vi "XLIN1.7-2048SQ TE0_Target.vi"() -> ()   [LabVIEW 2018]
uses:
  <vilib>/Platform/TimedLoop/XDataNode/timing_clust.ctl
  <vilib>/Platform/TimedLoop/XDataNode/nitl_modes.ctl
  <vilib>/Platform/TimedLoop/XDataNode/wakeup.ctl
  <vilib>/rvi/eio/common/nirviEmuTemplateMethod_errors.vi
  <vilib>/rvi/Emulation/niFpgaGetClockAttributes.vi
  <vilib>/rvi/Emulation/niFpgaSctlEmulationGetInTimedLoop.vi
  <vilib>/rvi/Emulation/niFpgaEmulationReportErrorSimple.vi
  <vilib>/rvi/Emulation/niFpgaProcessEmulError.vi
  <vilib>/rvi/Emulation/niFpgaCriticalErrorInLSC.vi
  <vilib>/rvi/interface/RandomDataEmulation/niFpgaRandomDataHandleErrors.vi
  <vilib>/eio/EIONode/EIONode.xnode
  <vilib>/Platform/TimedLoop/XDataNode/XDataNode.xnode
  <vilib>/rvi/DataTransferAndStorage/Container/XNode/niFpgaContainer.xnode
  <vilib>/rvi/interface/RandomDataEmulation/nirviRandomDataFpgaReadWriteTemplate.vi
  <vilib>/Platform/TimedLoop/XDataNode/XDNodeRunTimeDep.lvlib
panel:
  in  "SetFull":bool
  in  "GetCapture":bool
  in  "FIFO Enable = 0":u8
  in  "Ticks Reset = 7":u8=7
  in  "Tick Before Low CS":u64=1
  in  "Ticks After End Readout >0":u64=1
  in  "Ticks After ADC":u64
  in  "Stop FIFO Frame":u8=7
  in  "Output Data _ADCCLK(F) = 7":u8=7
  in  "True CDSCLK2 Stop = 5":u8=1
  in  "True CDSCLK2 Start = 4":u8
  in  "Ticks After Start Readout":u64=4
  in  "Ticks After Start Integration":u64
  in  "Ticks After Reset":u64
  in  "Ticks After Bot >0":u64=64
  in  "Ticks After Top >0":u64=64
  in  "Supply Select":u8(ring) items=["Local", "External"]
  in  "Counter R&F CLK_2 = 4":u8=4
  in  "F(F)/R(T)_CmAD":bool
  in  "Output Data _ADCCLK(T) = 3":u8=3
  in  "True ADCCLK Stop = 4":u8=4
  in  "True ADCCLK Start = 1":u8=1
  in  "Counter R&F CLK_1 = 7":u8=7
  in  "Falling CLK_2 = 2":u8=2
  in  "Rising CLK_2 = 1":u8=1
  in  "Falling CLK_1 = 1":u8=1
  in  "Rising CLK_1 = 0":u8
  in  "Counter R CLK = 2":u8=2
  in  "ResetFrame":bool
  in  "Data End Readout":u8[](array[numeric])=[0, 5, 1, 0, 0]
  in  "Command End Readout":u8[](array[numeric])=[8, 4, 2, 0, 0]
  in  "Data Start Readout":u8[](array[numeric])=[0, 0, 1, 11, 1, 0, 0, 0, 0, 6, 0, 0, 15, 0, 1, 3, 5, 13, 13, 0]
  in  "Command Start Readout":u8[](array[numeric])=[8, 4, 2, 2, 2, 2, 9, 2, 2, 2, 2, 2, 2, 1, 1, 1, 1, 1, 1, 0]
  in  "Data Start Integration":u8[](array[numeric])=[0, 0, 0, 1, 1, 0, 0, 0, 5, 1, 0, 0, 0, 0, 0, 0, 0, 0, 0, 0, 3, 1, 0, 0, 1, 5, 1, 0, 0, 1, 3, 1, 0, 0, 1, 3, 1, 0, 0, 1, 11, 1, 11, 0, 1, 11, 1, 3, 0, 0, 0]
  in  "Command Start Integration":u8[](array[numeric])=[8, 4, 2, 2, 2, 2, 9, 2, 2, 2, 2, 2, 0, 0, 0, 0, 0, 8, 4, 2, 2, 2, 2, 9, 2, 2, 2, 2, 9, 2, 2, 2, 2, 9, 2, 2, 2, 2, 9, 2, 2, 2, 2, 9, 2, 2, 2, 2, 9, 0, 0]
  in  "Data Reset":u8[](array[numeric])=[0, 0, 0, 5, 0, 0, 0, 0]
  in  "Command Reset":u8[](array[numeric])=[8, 4, 2, 2, 2, 2, 9, 0]
  in  "IN1":bool
  in  "IN2":bool
  in  "RS":bool
  in  "1032 pixels":u16=1032
  in  "Pixel (n-3) = 3":u16=3
  in  "R MCLK = 2":u16=2
  in  "Command array":bool[](array[boolean])=[FALSE, FALSE, FALSE, FALSE, FALSE, FALSE, FALSE, FALSE, FALSE, FALSE, FALSE, FALSE, FALSE, FALSE, FALSE, FALSE, FALSE]
  in  "Read(T)/Write(F)":bool
  in  "Enum":T1(ring)=enum."GREEN PGA"
  in  "Write Data":bool[](array[boolean])=[FALSE, FALSE, FALSE, FALSE, FALSE, FALSE, FALSE, FALSE, FALSE]
  out "READ":bool[](array[boolean])
  in  "Конфигурация":bool
  out "FrameIsDone":bool
  in  "NumberOfAddFIFO":u16=2064
  in  "7..0(F)/0..7(T)":bool
  out "FIFOCounter":u16
  in  "Data CSBot":u8[](array[numeric])=[0, 9, 8, 11, 0, 6, 0, 2, 11, 0, 8, 0, 0, 0, 0, 9, 1, 3, 11, 7, 15, 15, 5, 15, 0, 1, 15, 15, 5, 8, 5, 2, 3, 0, 8, 2, 3, 3, 3, 3, 3, 3, 3, 2, 0]
  in  "Автомат":bool
  in  "Data CSTop":u8[](array[numeric])=[0, 9, 12, 11, 0, 6, 0, 2, 11, 0, 8, 0, 0, 0, 0, 9, 1, 3, 3, 7, 15, 15, 5, 15, 0, 1, 15, 15, 5, 8, 5, 2, 3, 0, 8, 2, 3, 3, 3, 3, 3, 3, 3, 2, 0]
  in  "Command CS":u8[](array[numeric])=[8, 4, 2, 2, 2, 2, 2, 2, 2, 2, 2, 2, 2, 2, 2, 2, 2, 2, 2, 2, 2, 2, 2, 2, 2, 2, 2, 2, 2, 2, 2, 2, 2, 8, 4, 1, 1, 1, 1, 1, 1, 1, 1, 1, 0]
  in  "Stop_FPGA":bool
  in  "SetPreCapture":bool
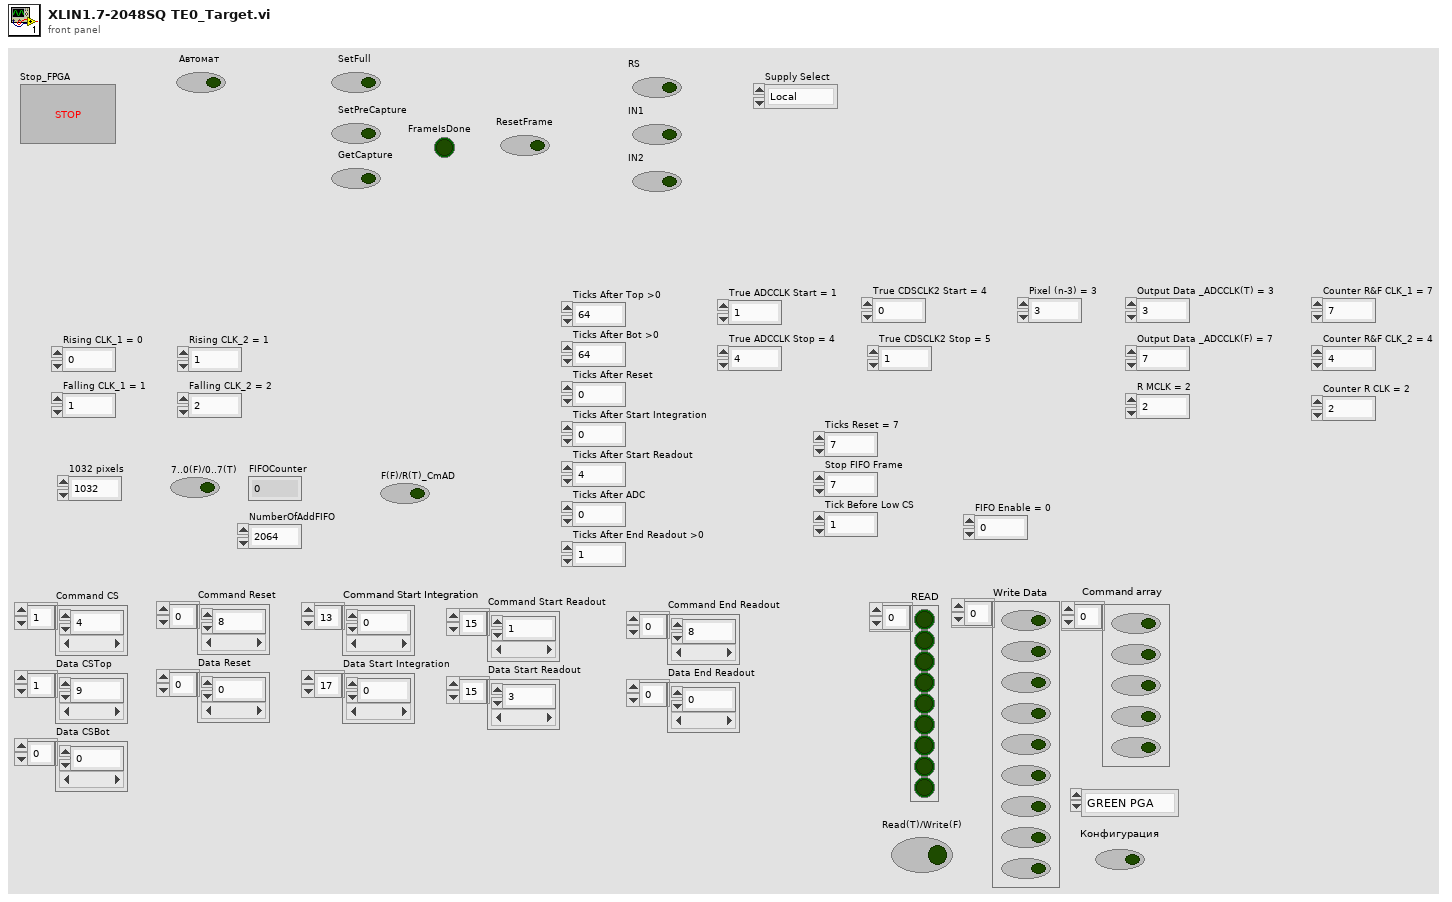
[diagram p1: front panel]
types:
  T1 = enum16{"Configuration", "MUX", "RED PGA", "GREEN PGA", "BLUE PGA", "RED OFF", "GREEN OFF", "BLUE OFF"}
  T2 = typedef "XDNodeRunTimeDep.lvlib/timing_clust.ctl" = cluster{"Expected End [f-1]":u64, "Actual End [f-1]":u64, "Finished Late? [f-1]":bool, "Expected End [i-1]":u64, "Actual End [i-1]":u64, "Finished Late? [i-1]":bool, "Expected Start [i]":u64, "Actual Start [i]":u64, "Expected Start [f]":u64, "Actual Start [f]":u64, "Source Name":string, "Structure Name":string, "Period":i64, "Deadline":i64, "Offset":i64, "Start":i64, "Priority":i32, "Timeout":i32, "Mode":T3, "Wakeup Reason":T4, "Error":errorcluster, "Source Type":string, "Secondary Source Type":string, "Global End Time":u64, "Global Start Time":u64, "Frame Duration":u64, "Iteration Duration":u64, "Assigned CPU":i32, "I/O Scan Engine Mode":u32}
  T3 = typedef "XDNodeRunTimeDep.lvlib/nitl_modes.ctl" = enum32{"No Change", "Process missed periods, maintain original phase", "Discard missed periods, maintain original phase", "Process missed periods, ignore original phase", "Discard missed periods, ignore original phase"}
  T4 = typedef "XDNodeRunTimeDep.lvlib/wakeup.ctl" = enum32{"Normal", "Aborted", "Asynchronous wakeup", "Timing source error", "Timed loop error", "Timeout"}
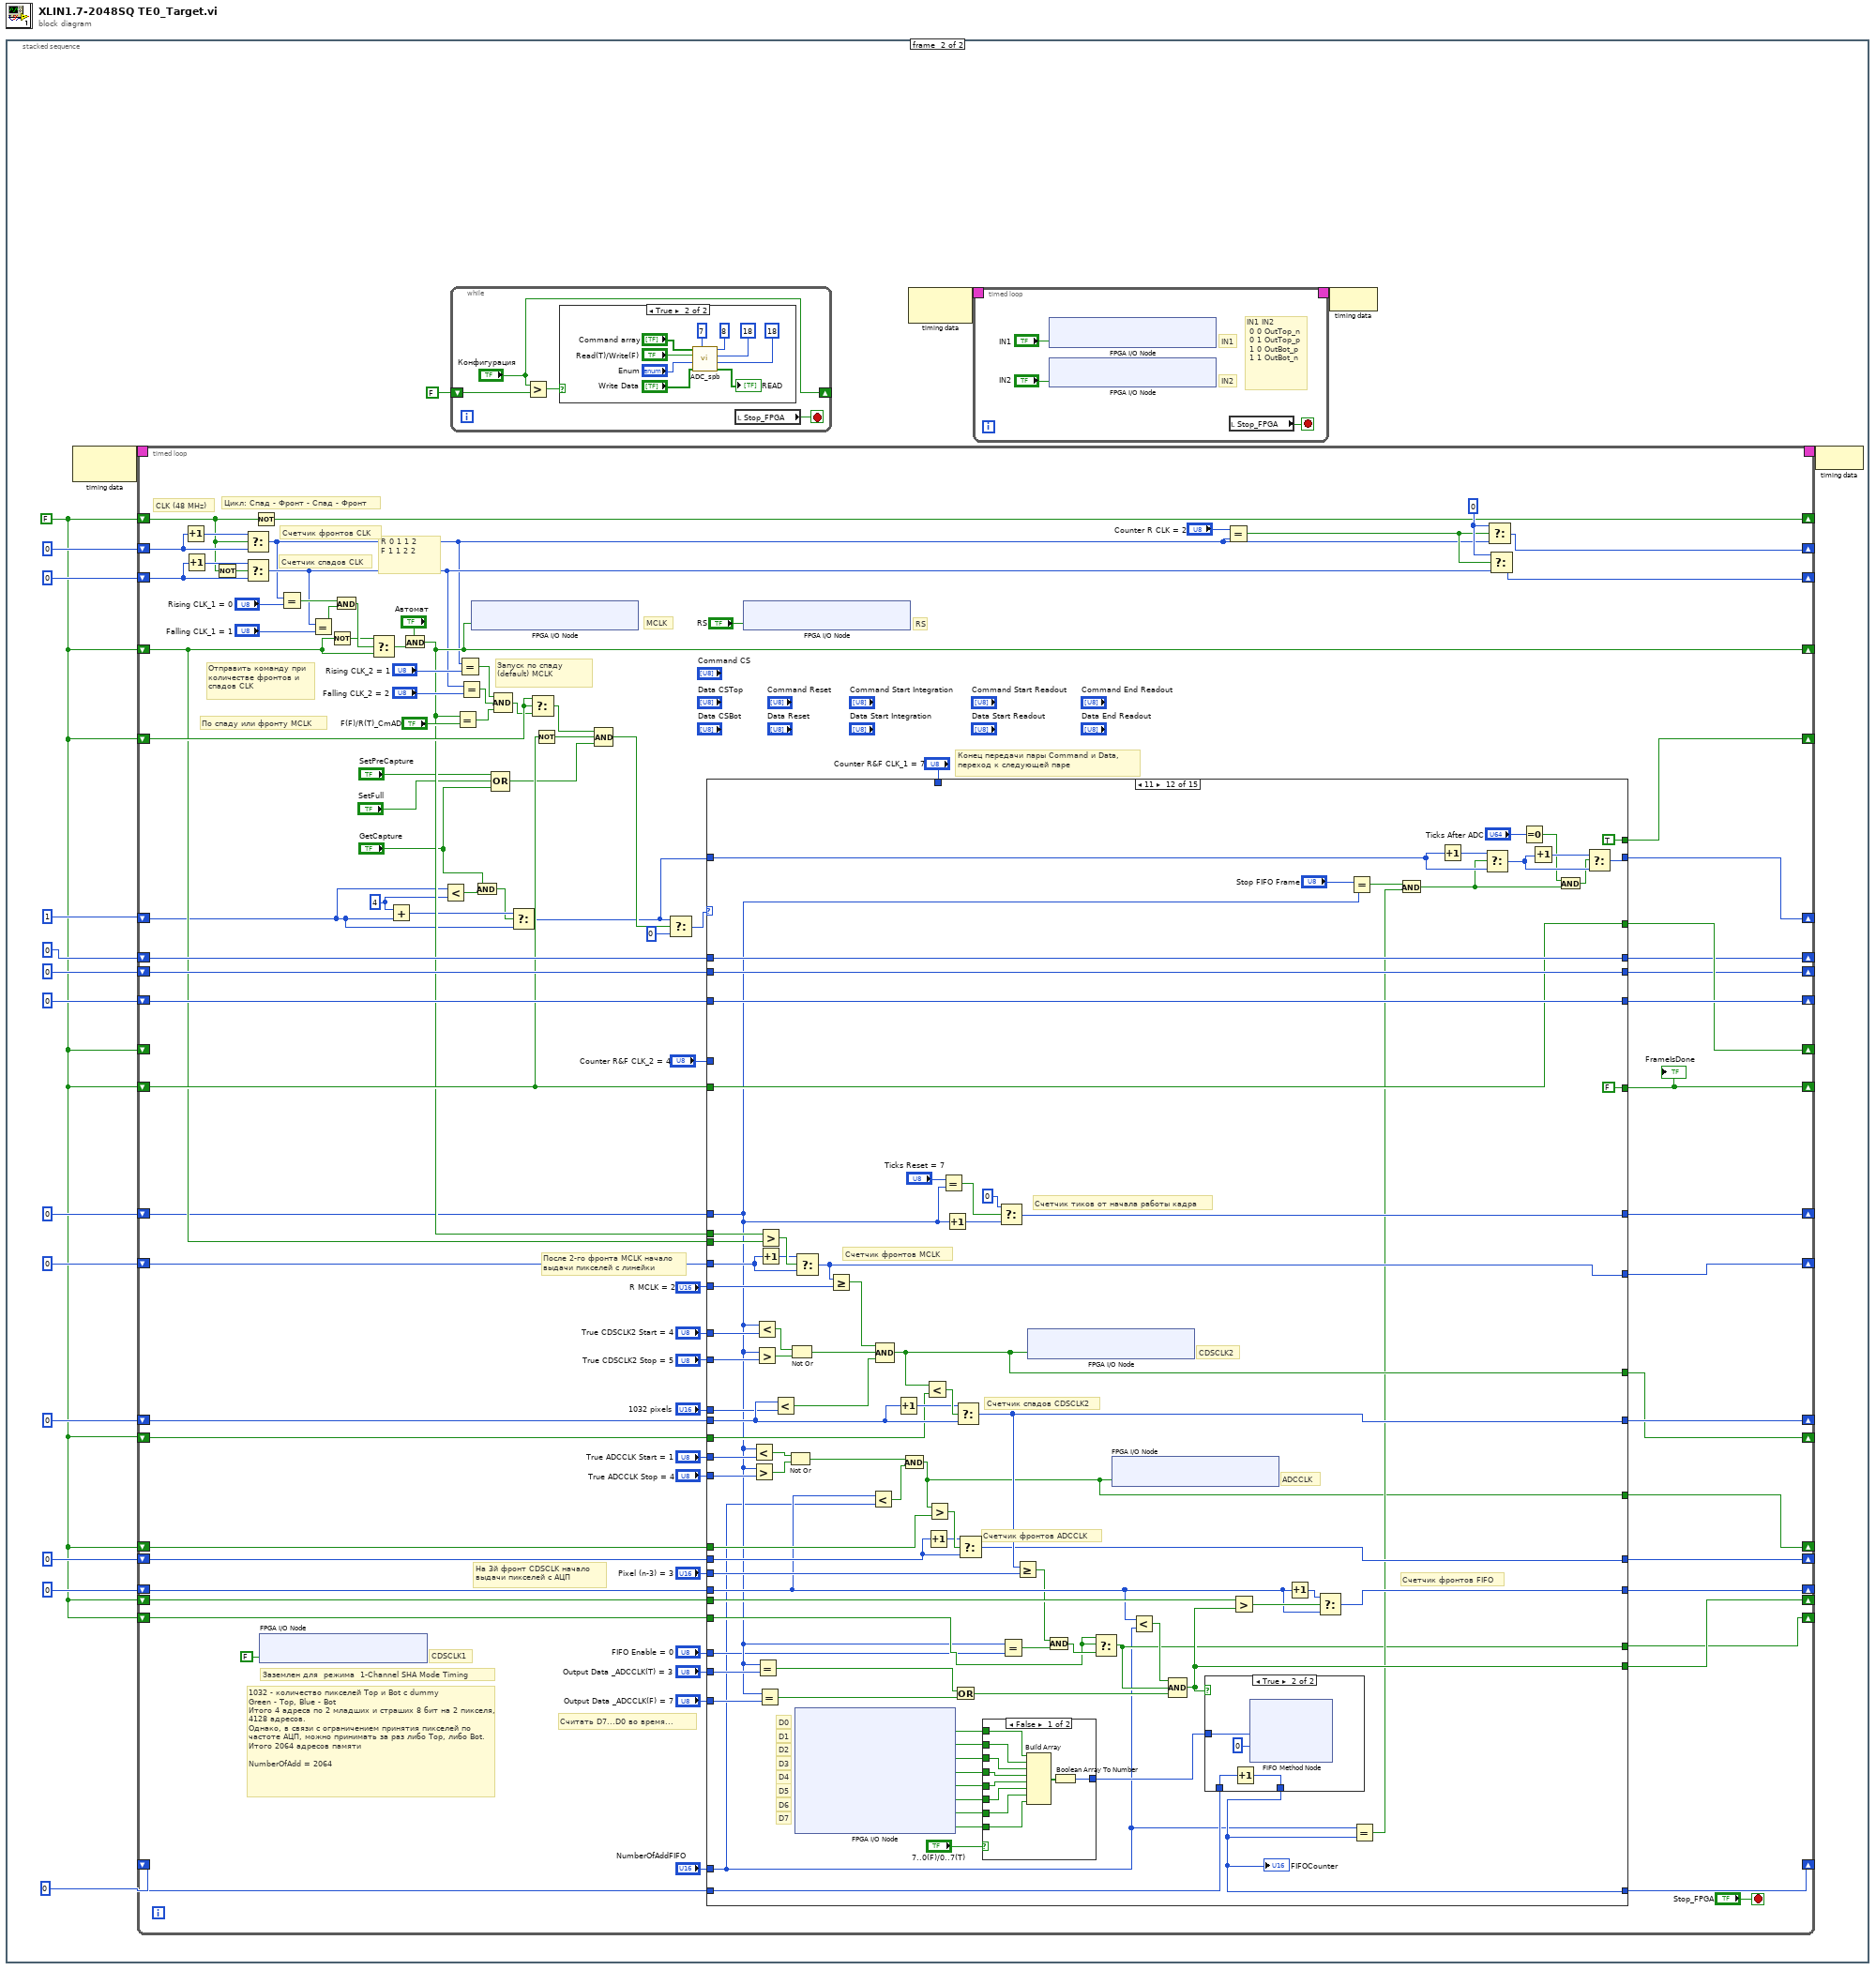
[diagram p0: block diagram]
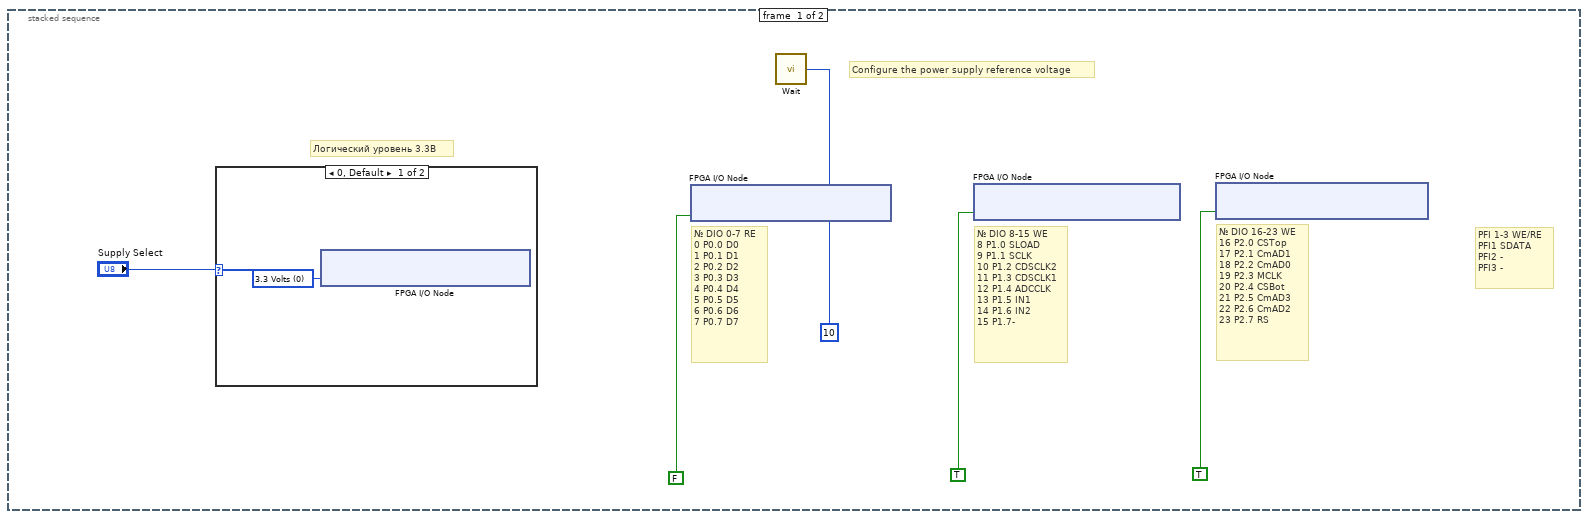
[diagram p2: hidden frame]
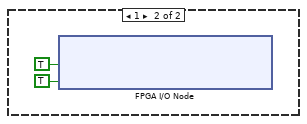
[diagram p3: hidden frame]
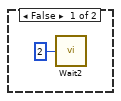
[diagram p4: hidden frame]
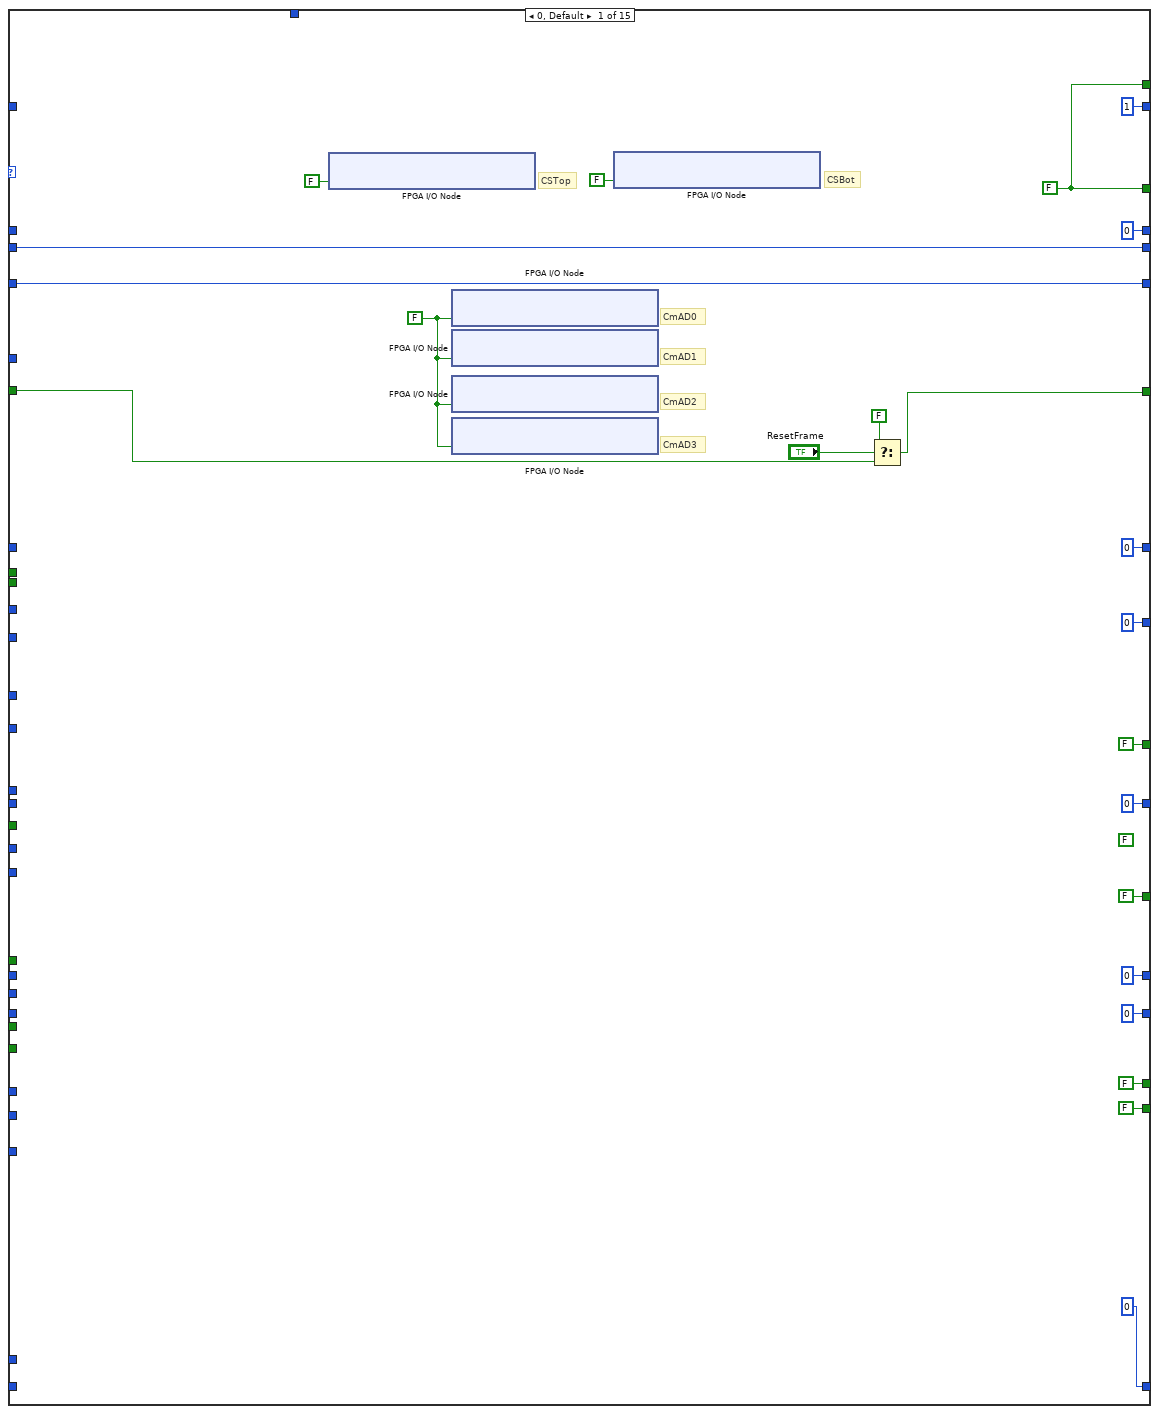
[diagram p5: hidden frame]
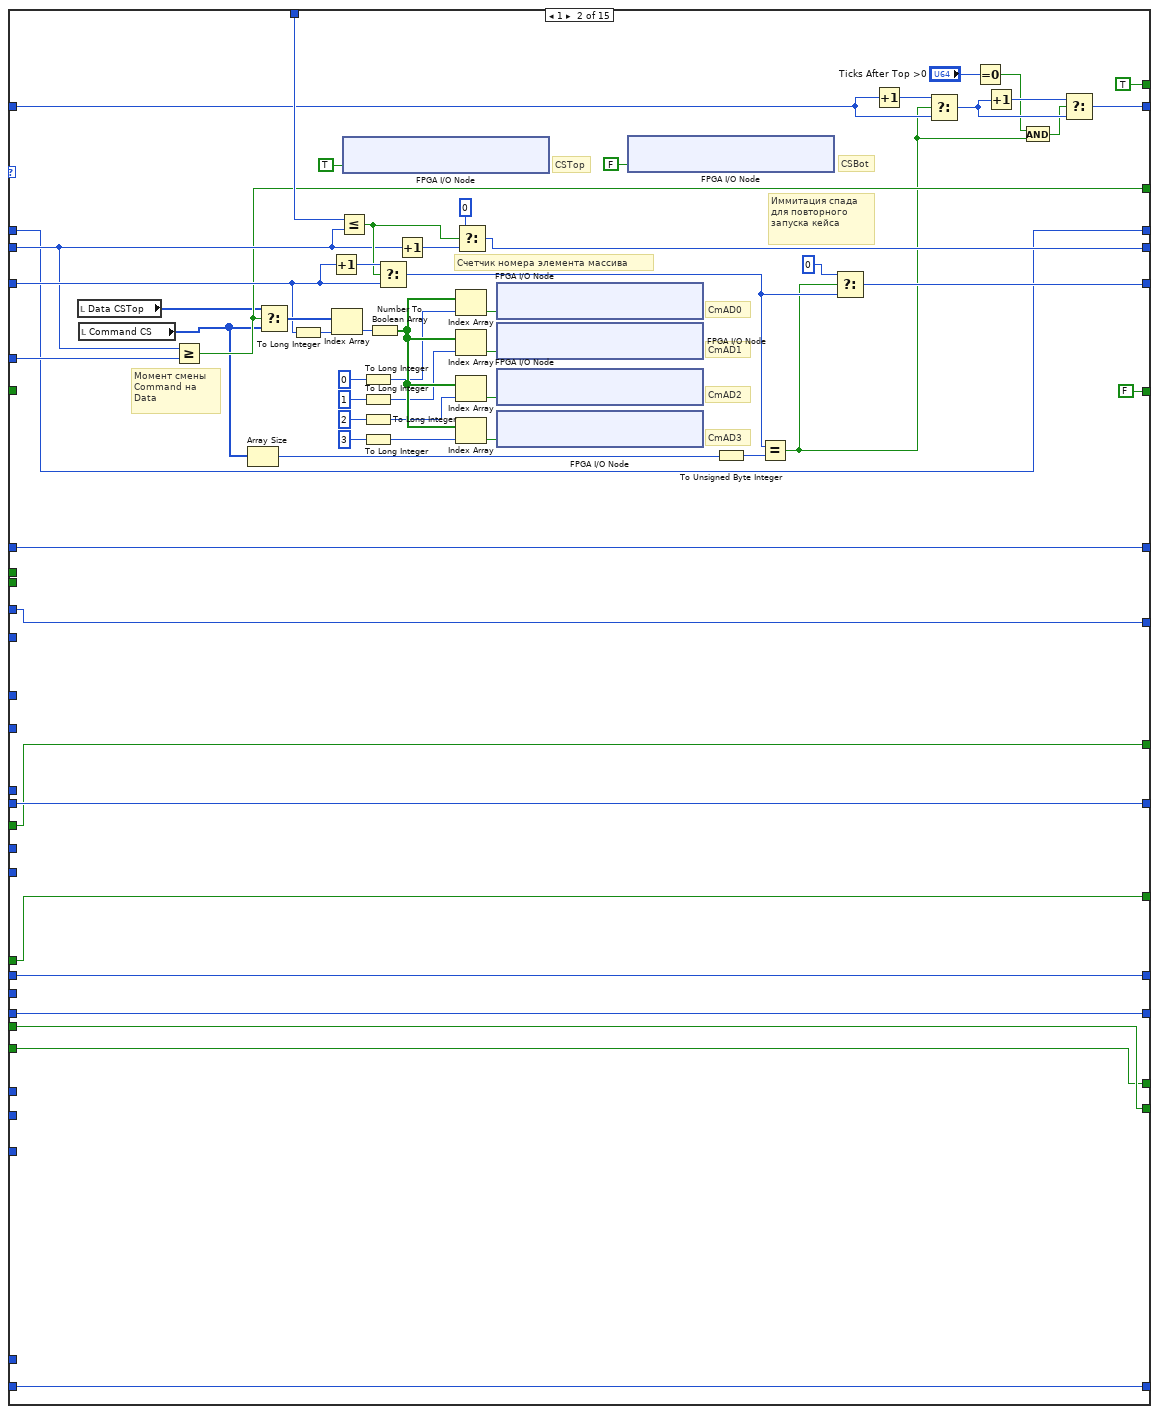
[diagram p6: hidden frame]
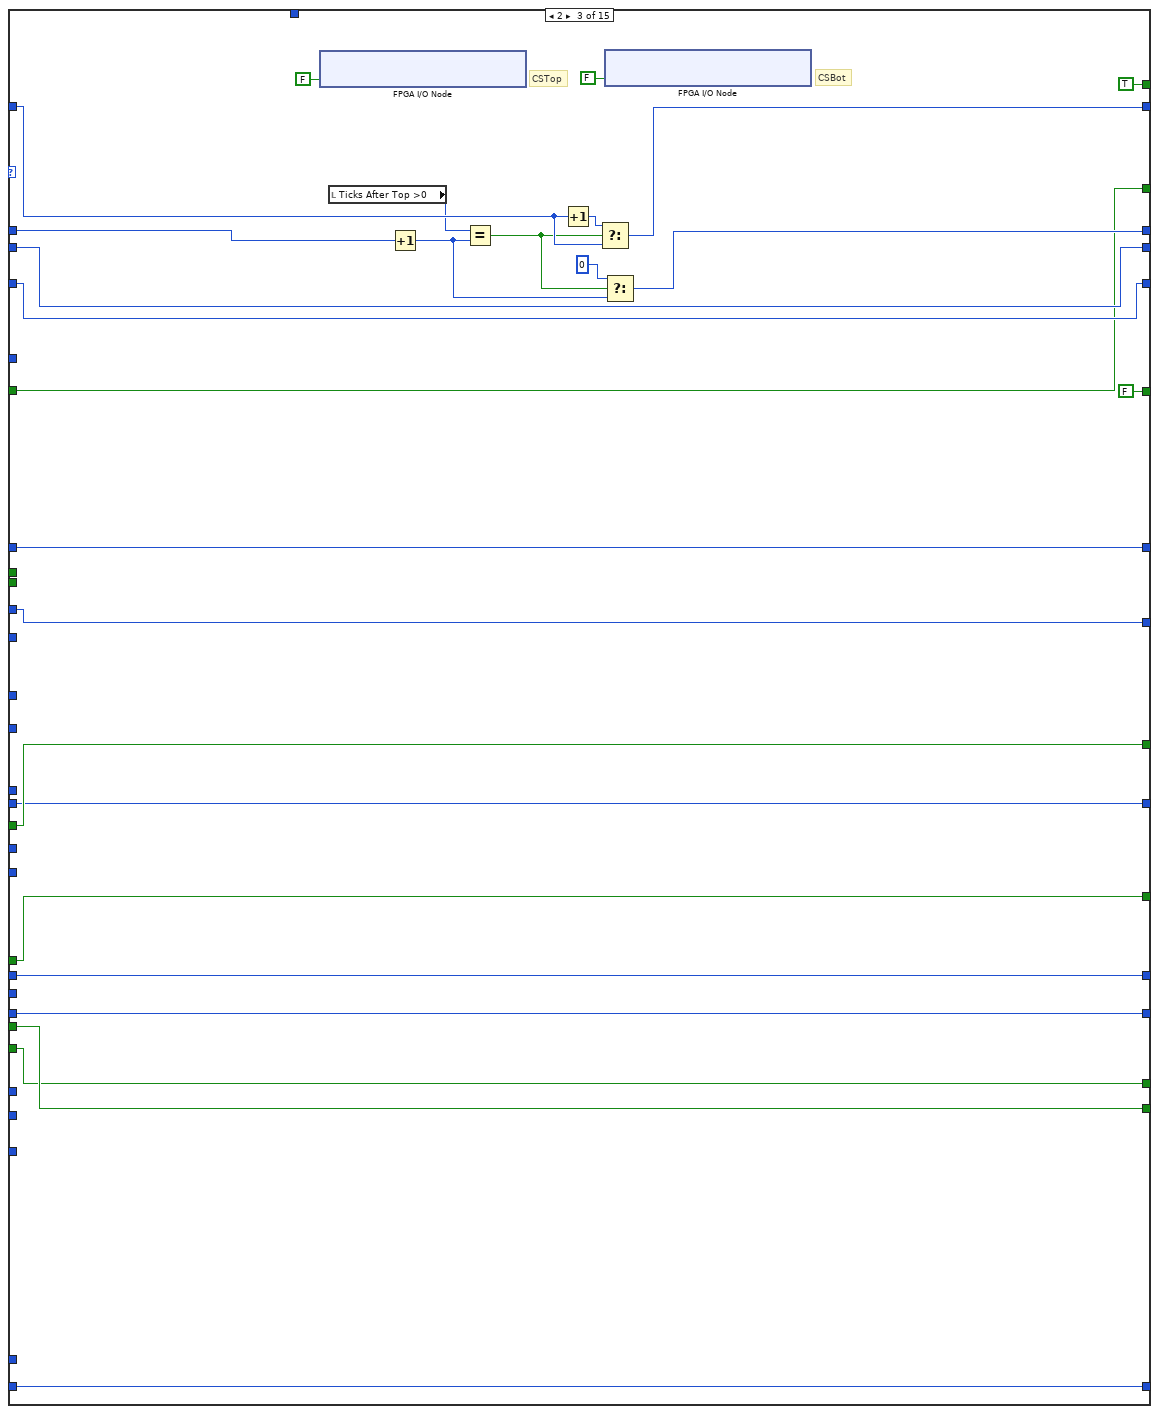
[diagram p7: hidden frame]
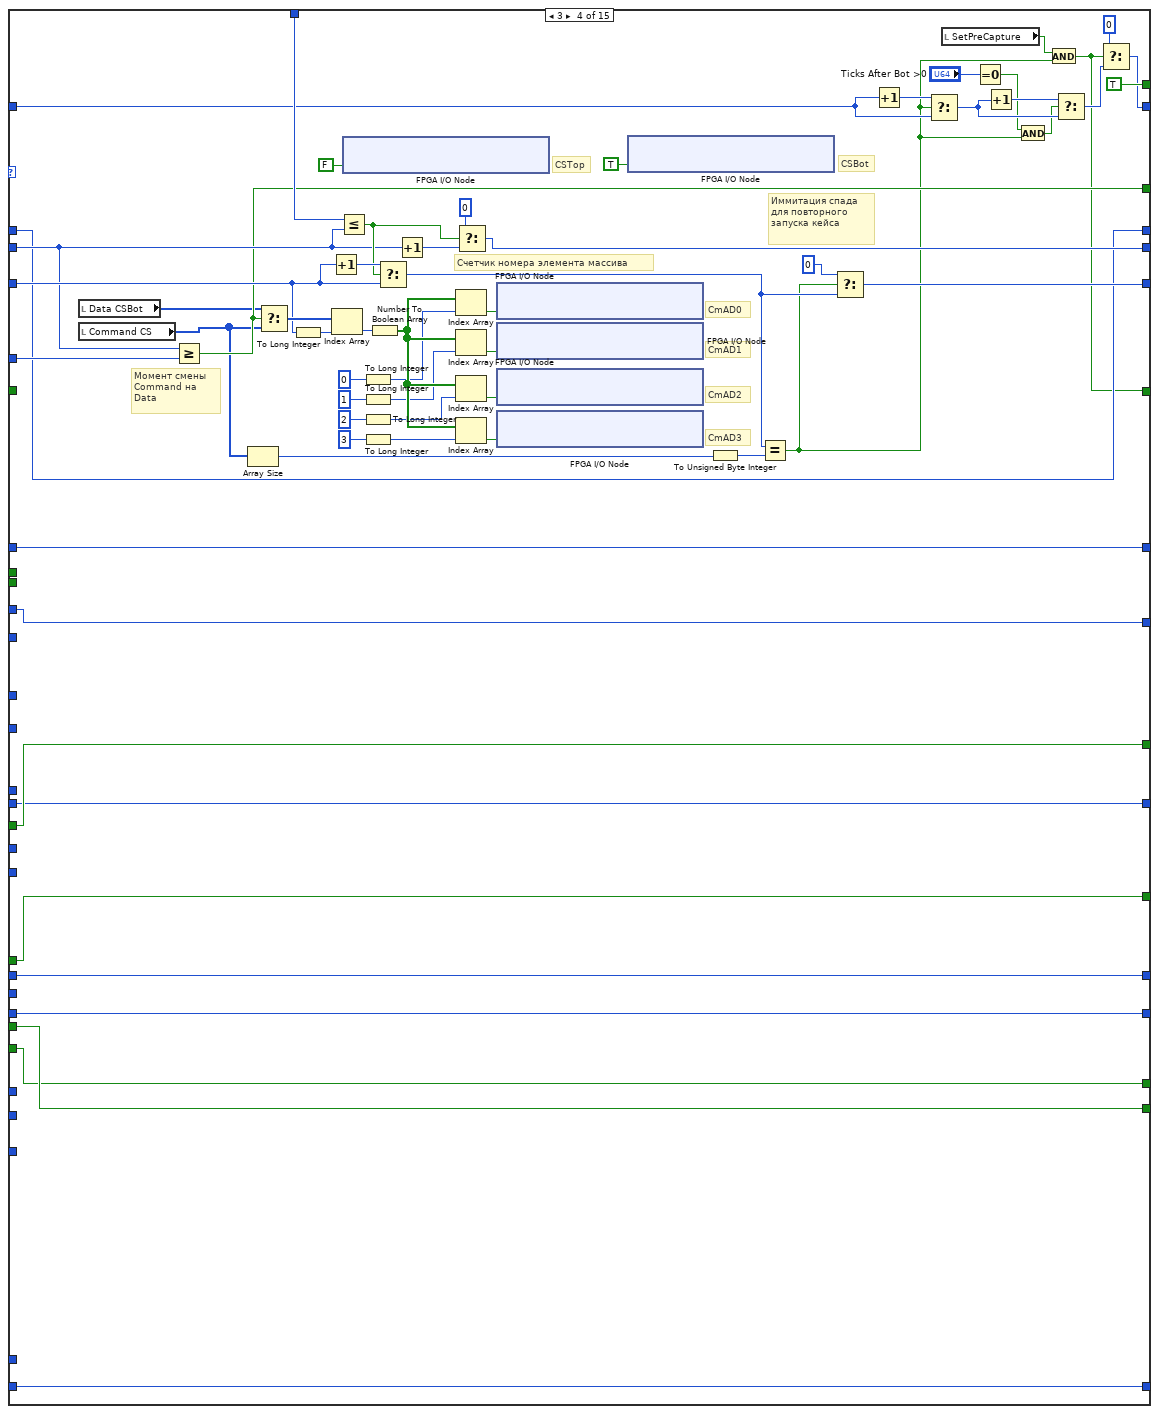
[diagram p8: hidden frame]
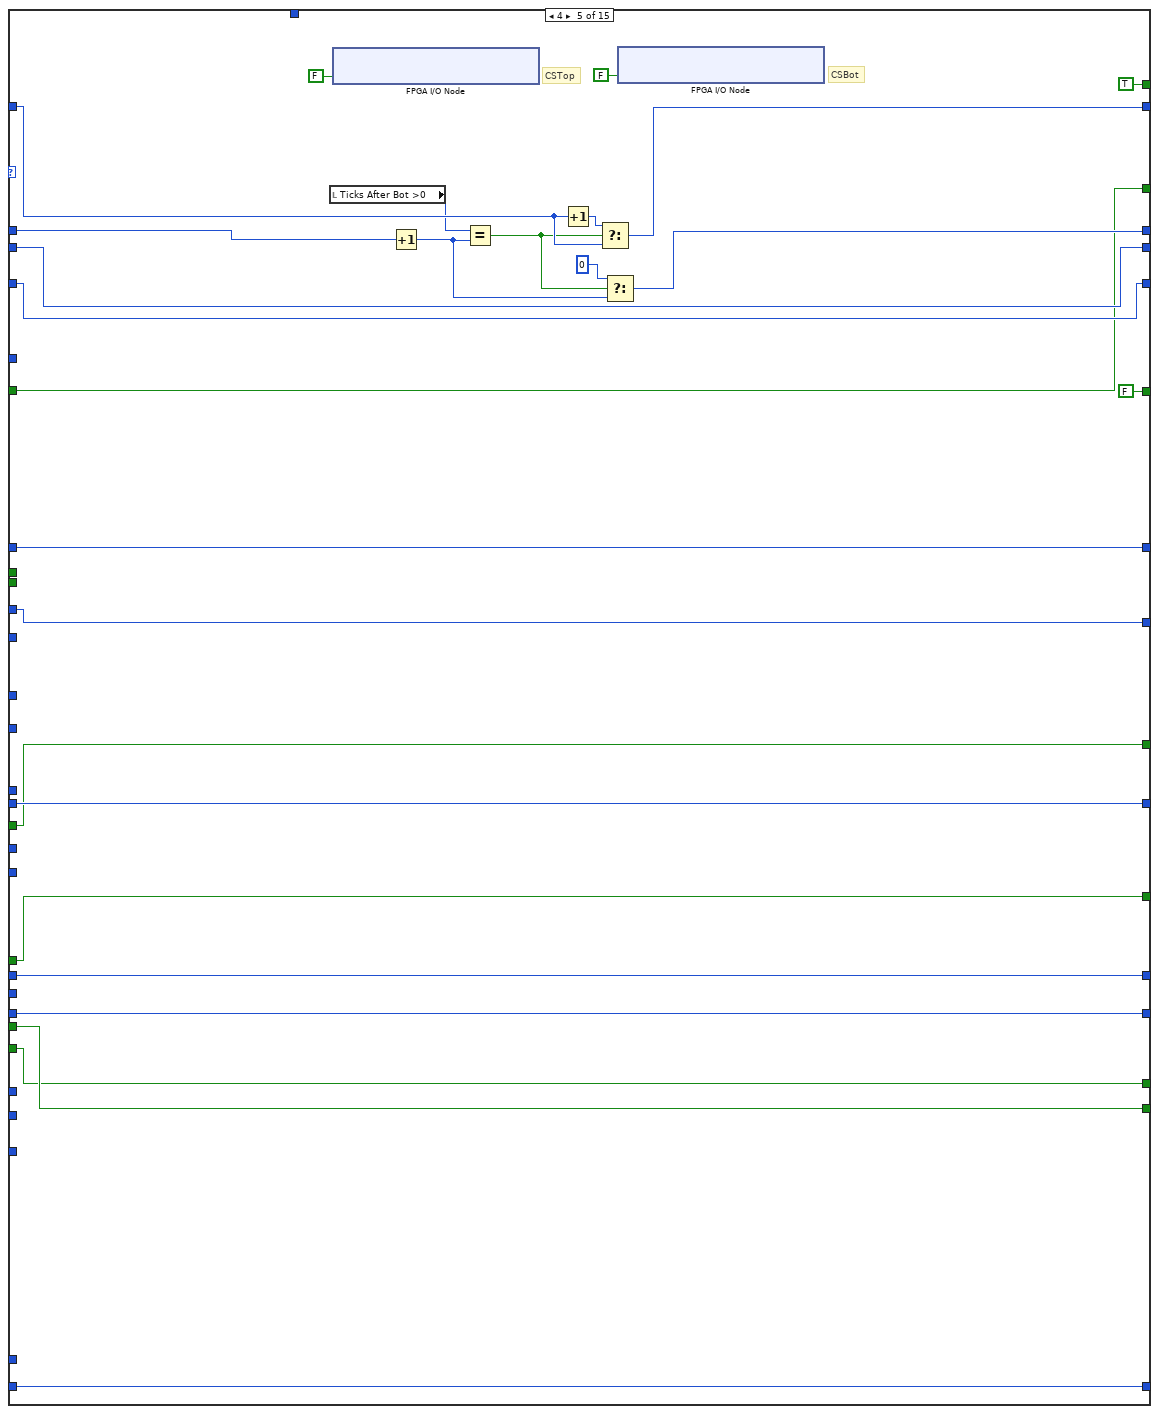
[diagram p9: hidden frame]
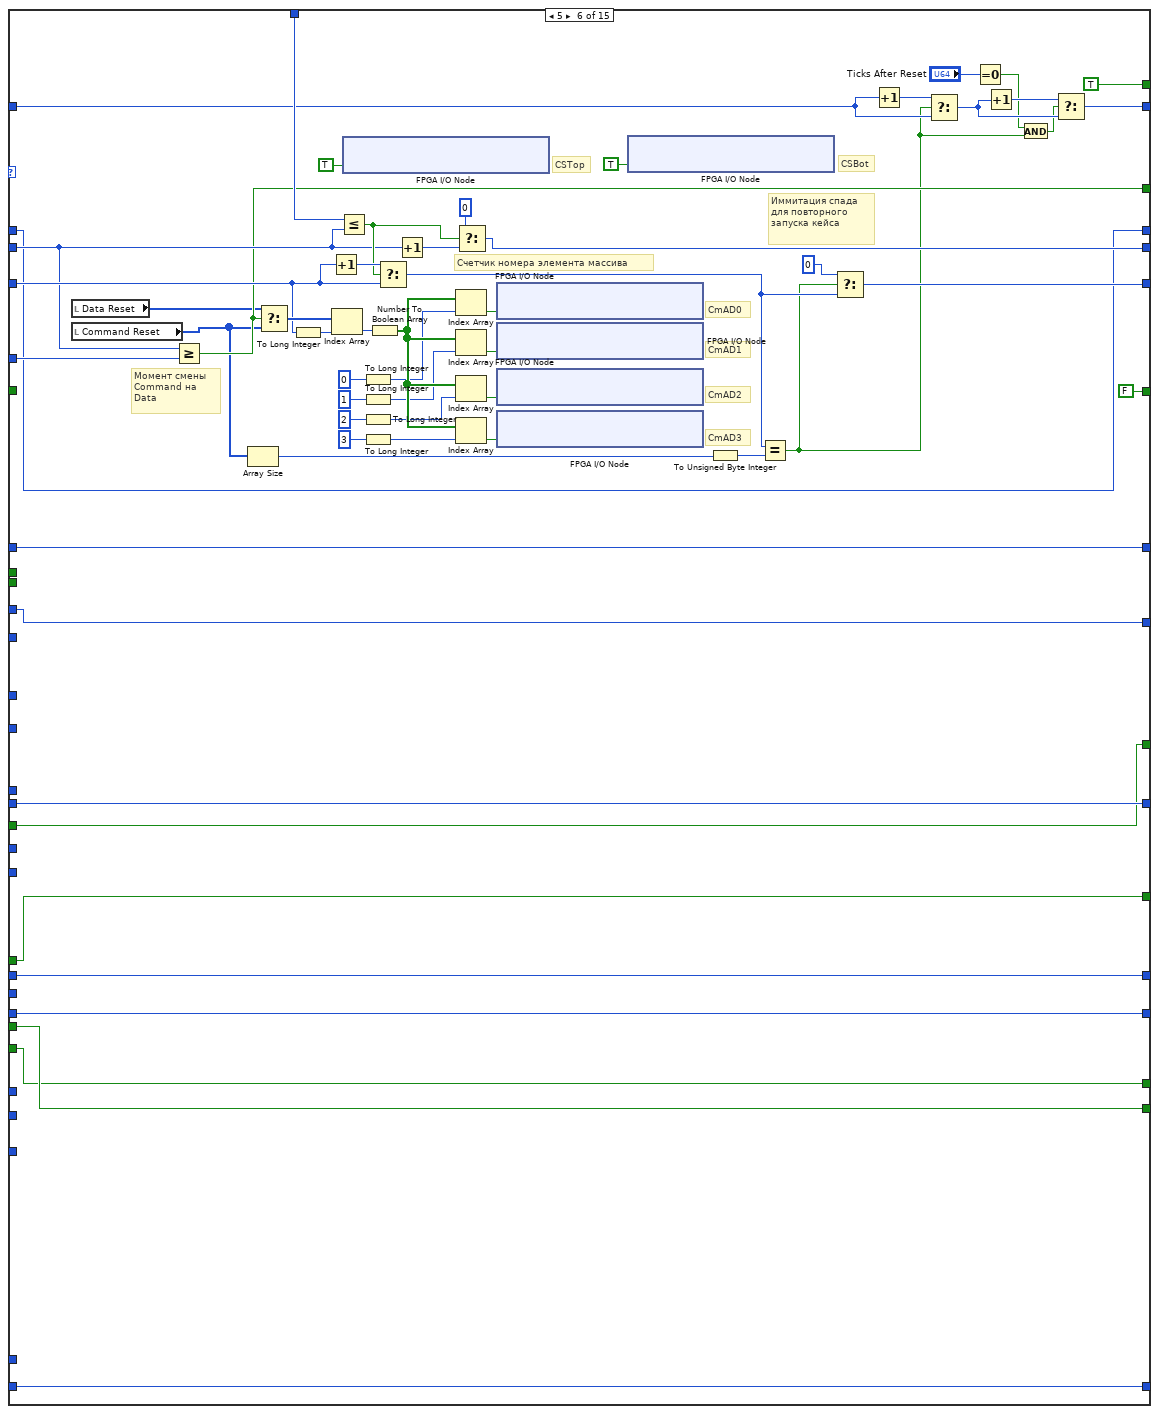
[diagram p10: hidden frame]
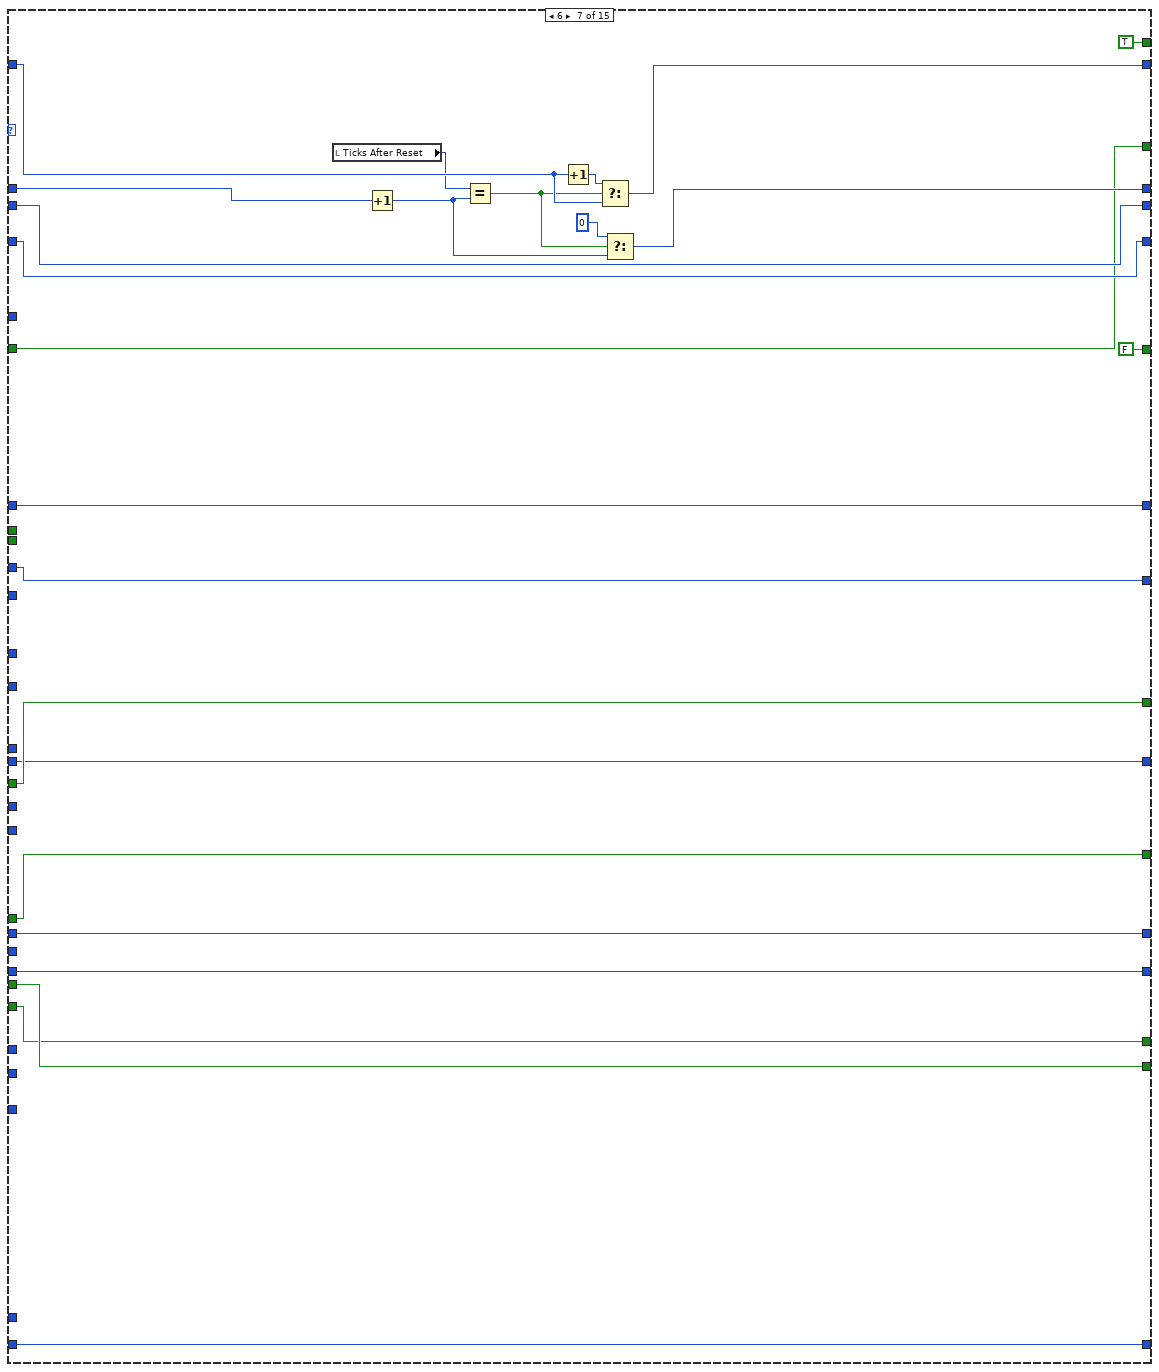
[diagram p11: hidden frame]
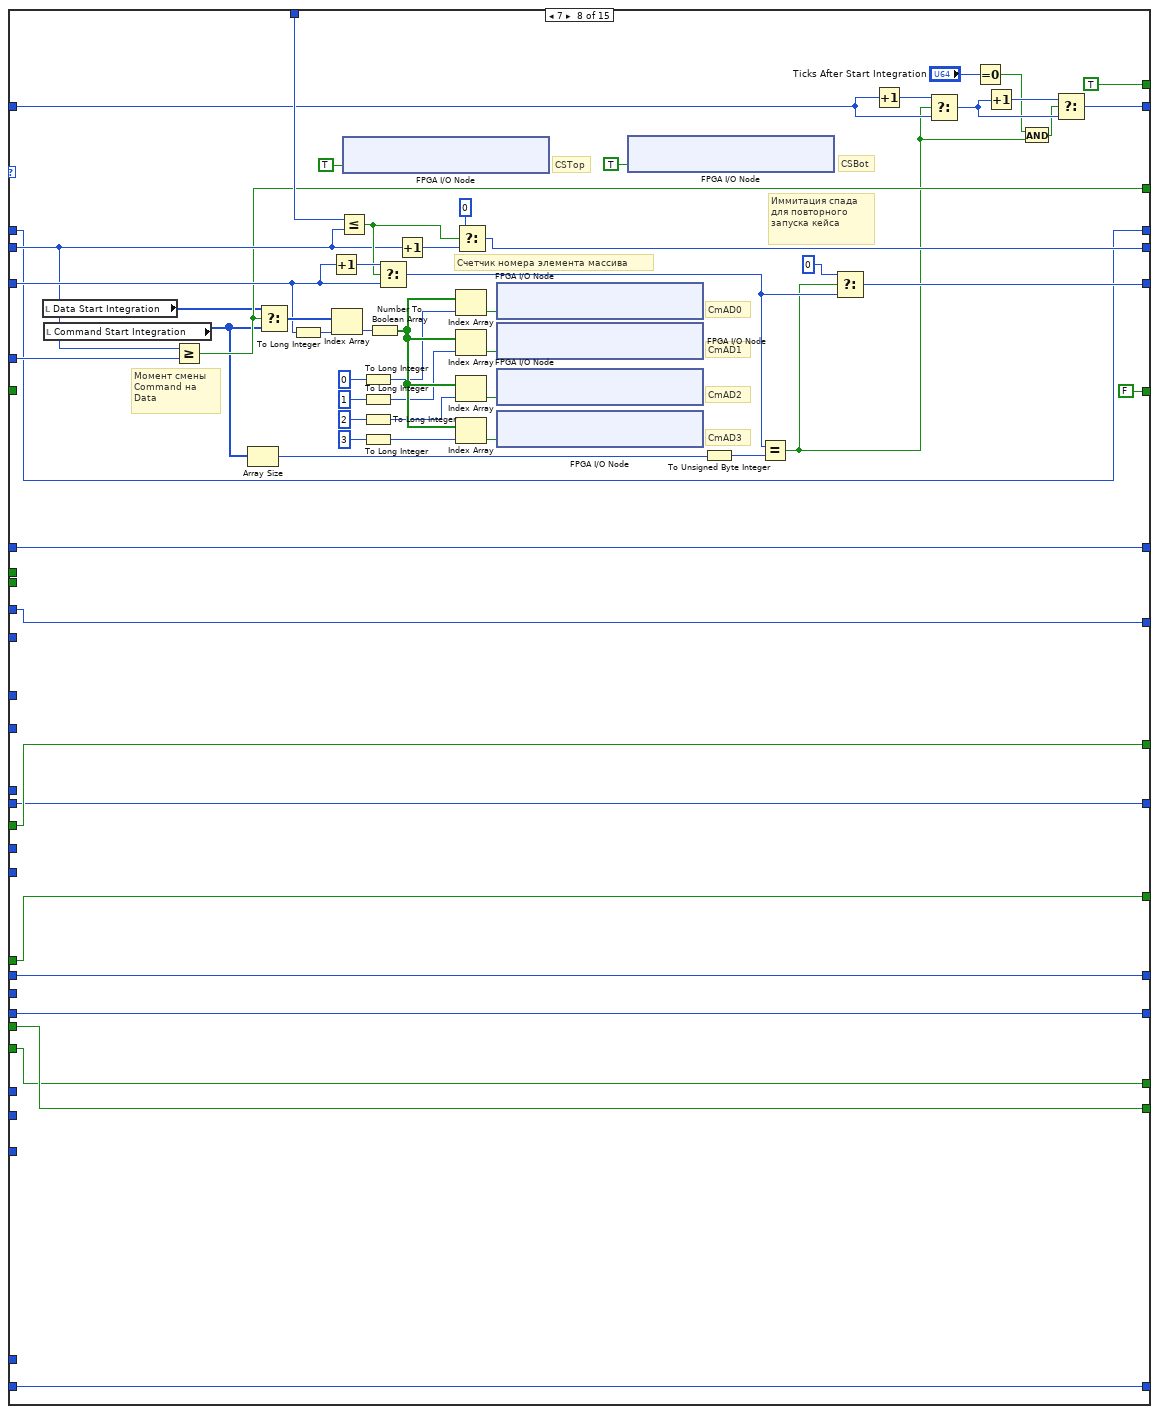
[diagram p12: hidden frame]
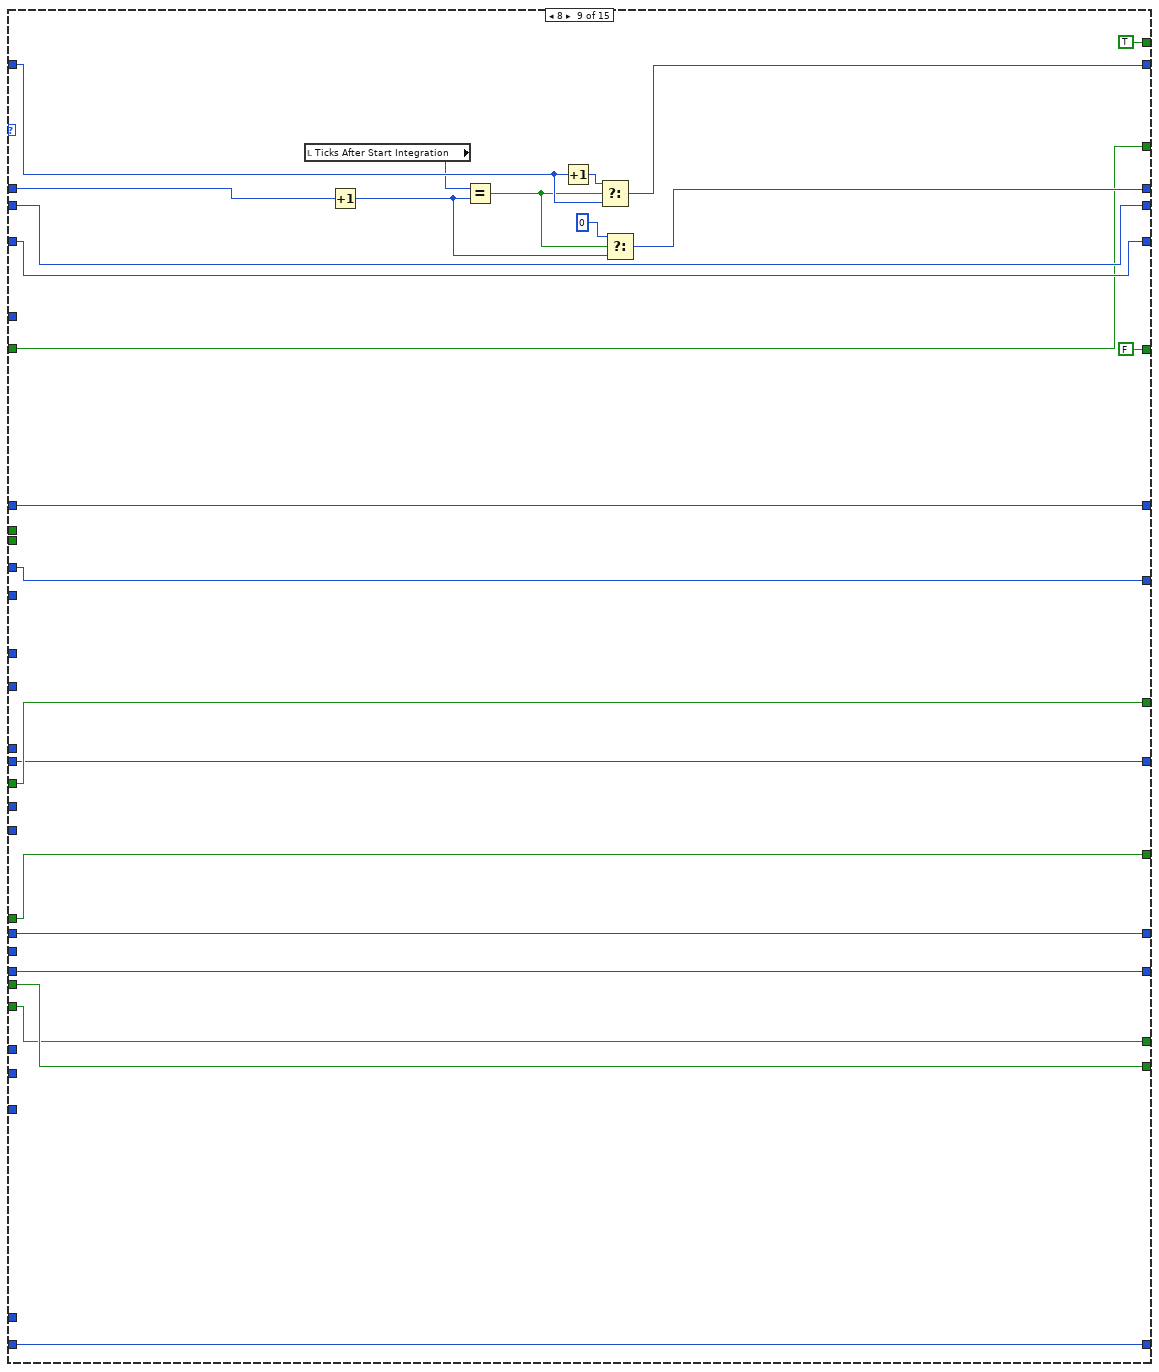
[diagram p13: hidden frame]
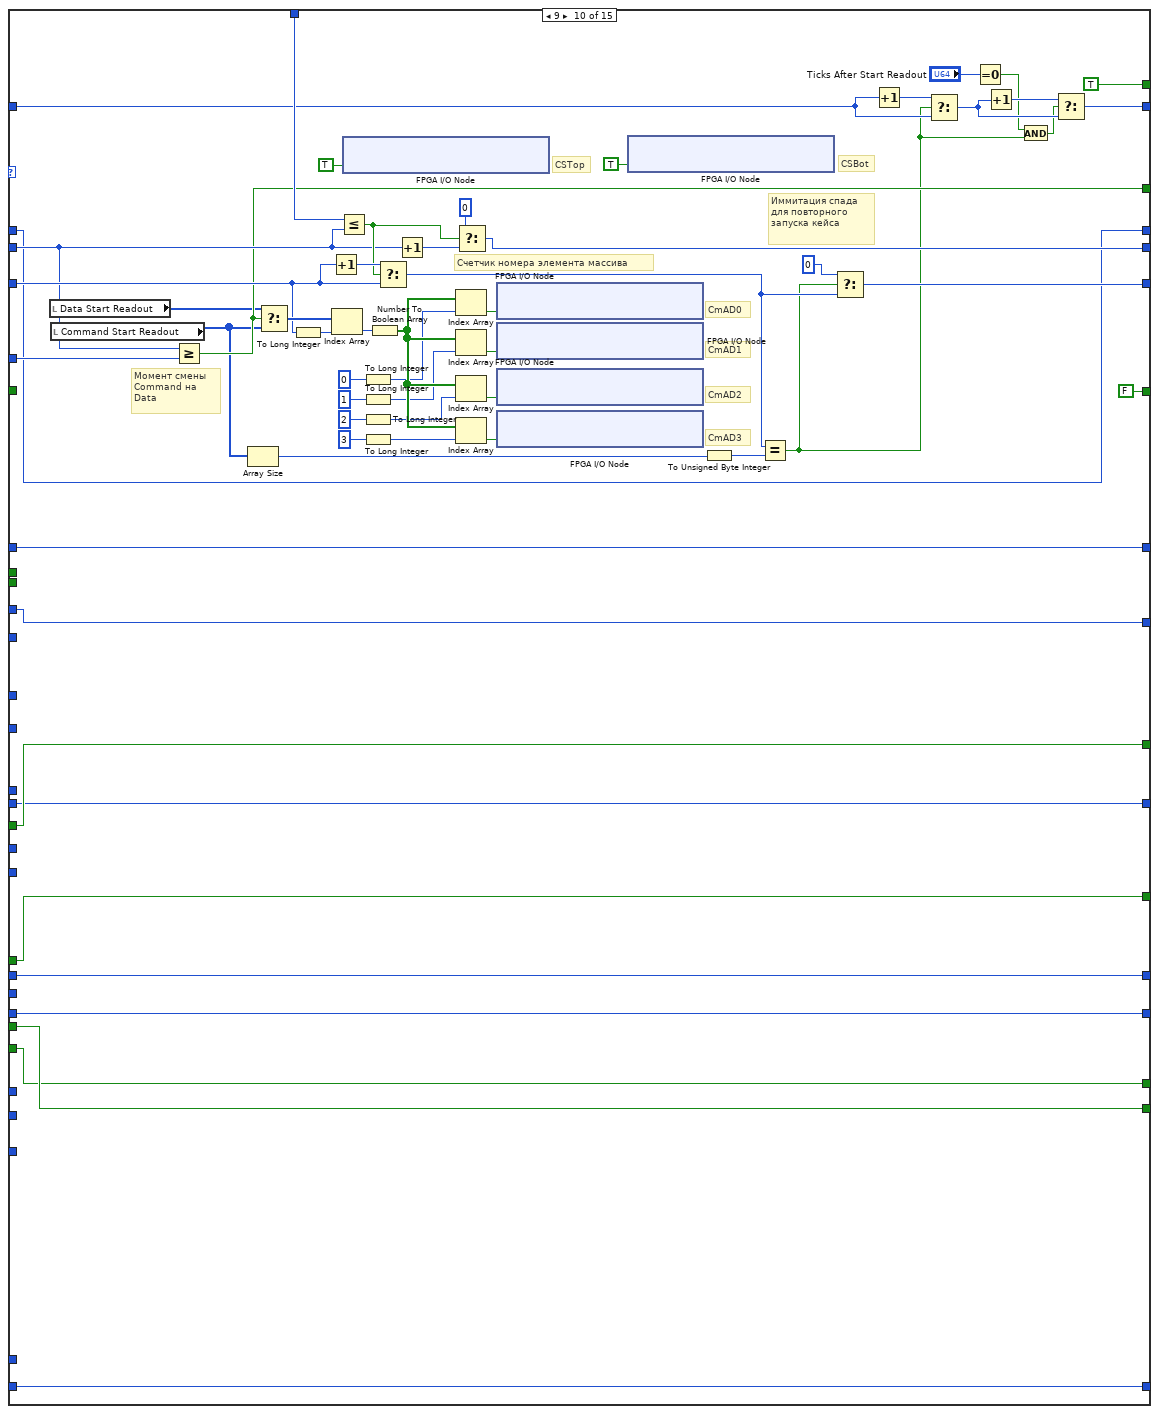
[diagram p14: hidden frame]
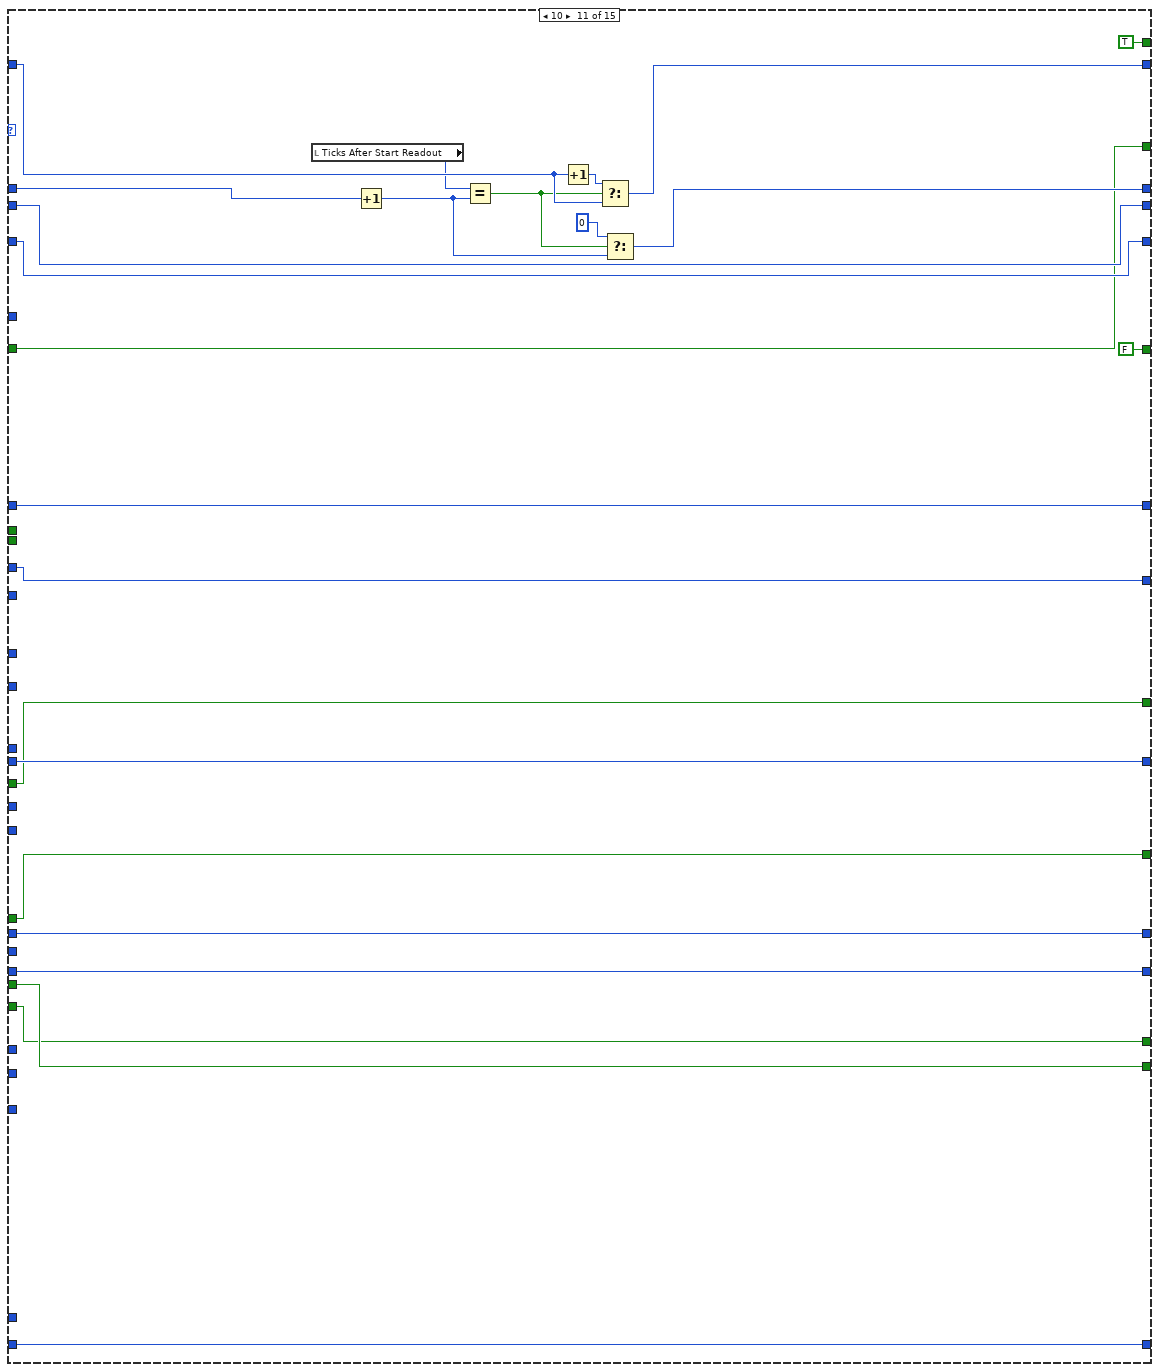
[diagram p15: hidden frame]
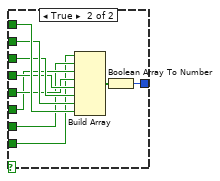
[diagram p16: hidden frame]
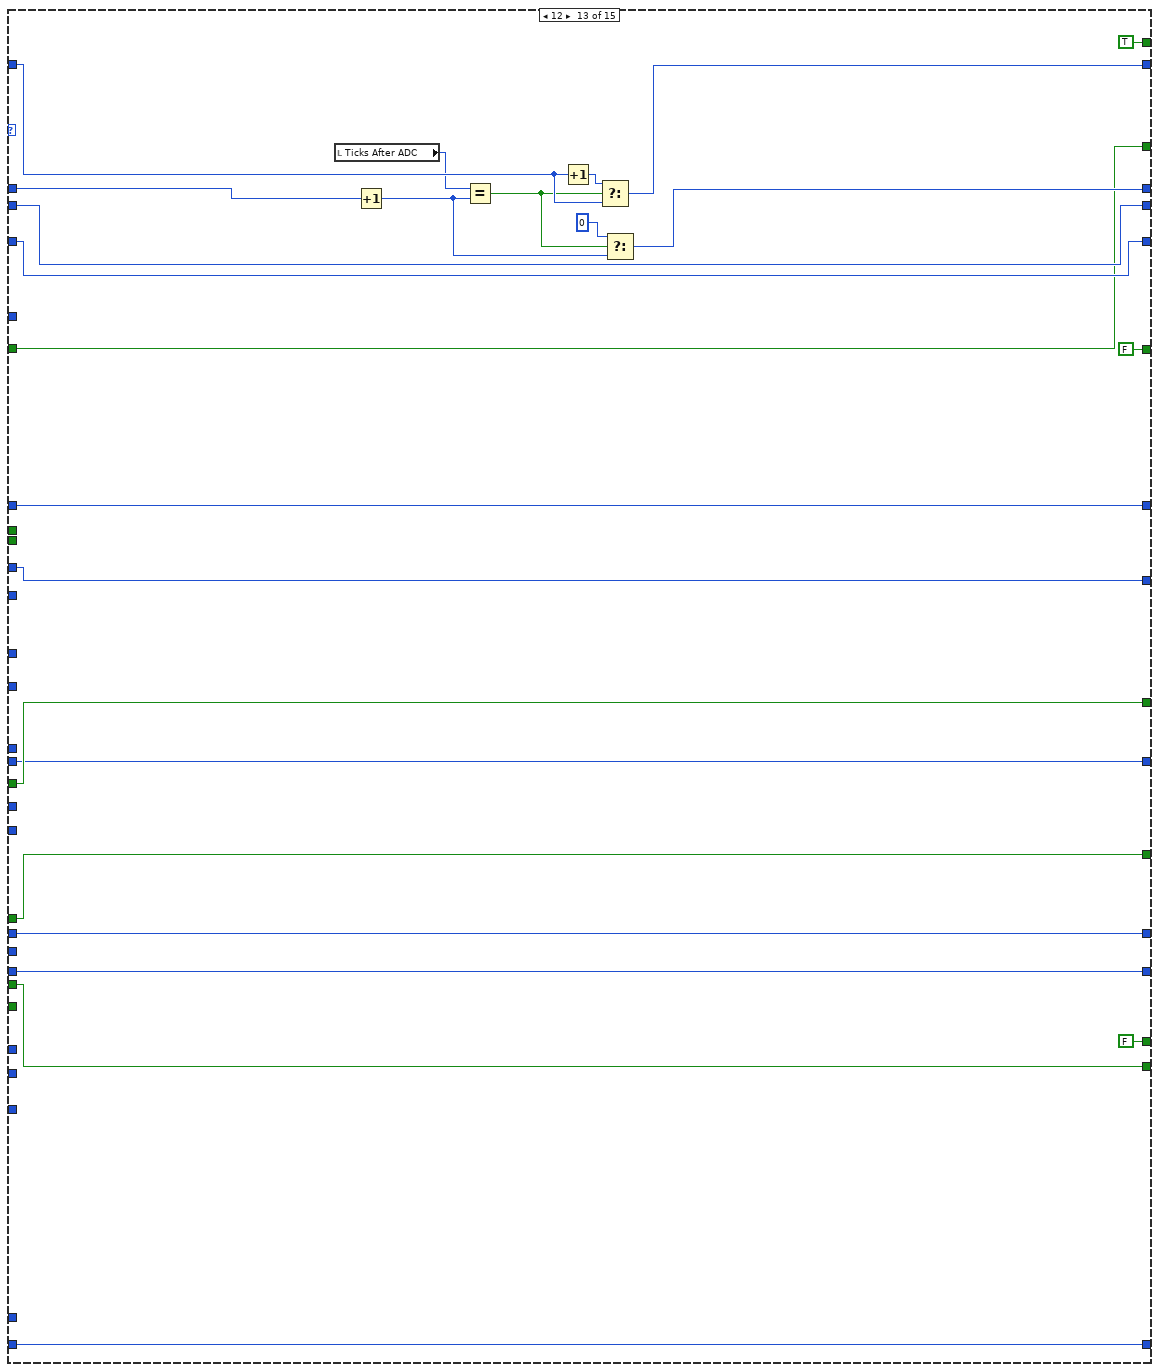
[diagram p18: hidden frame]
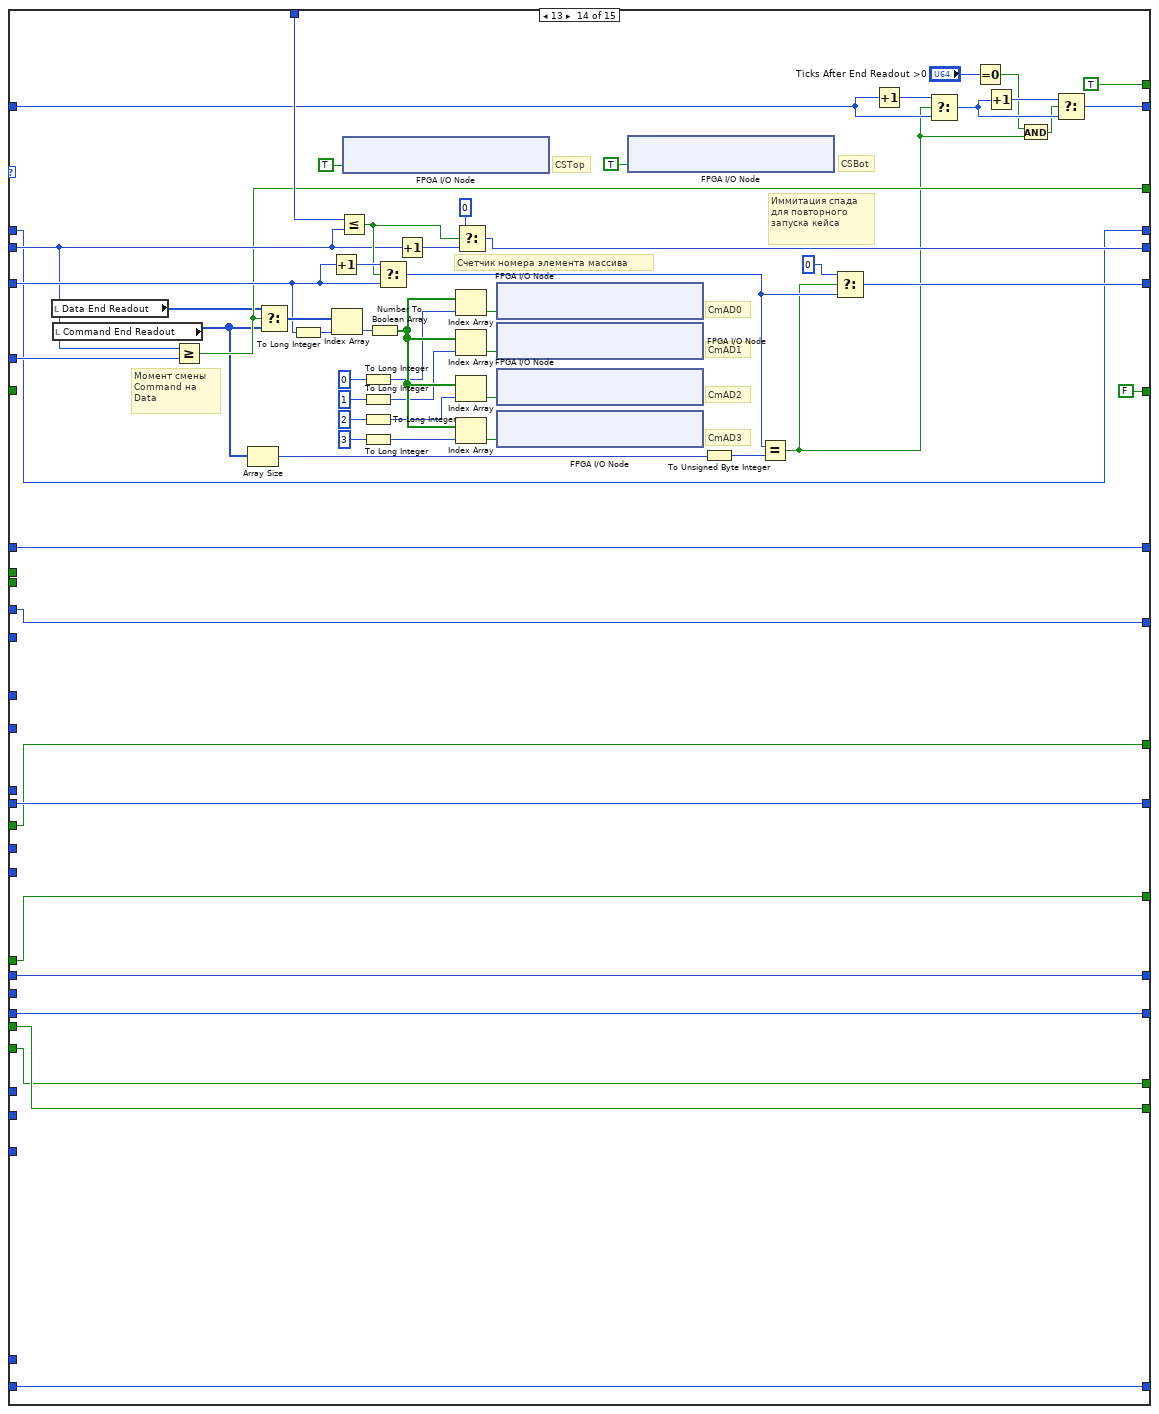
[diagram p19: hidden frame]
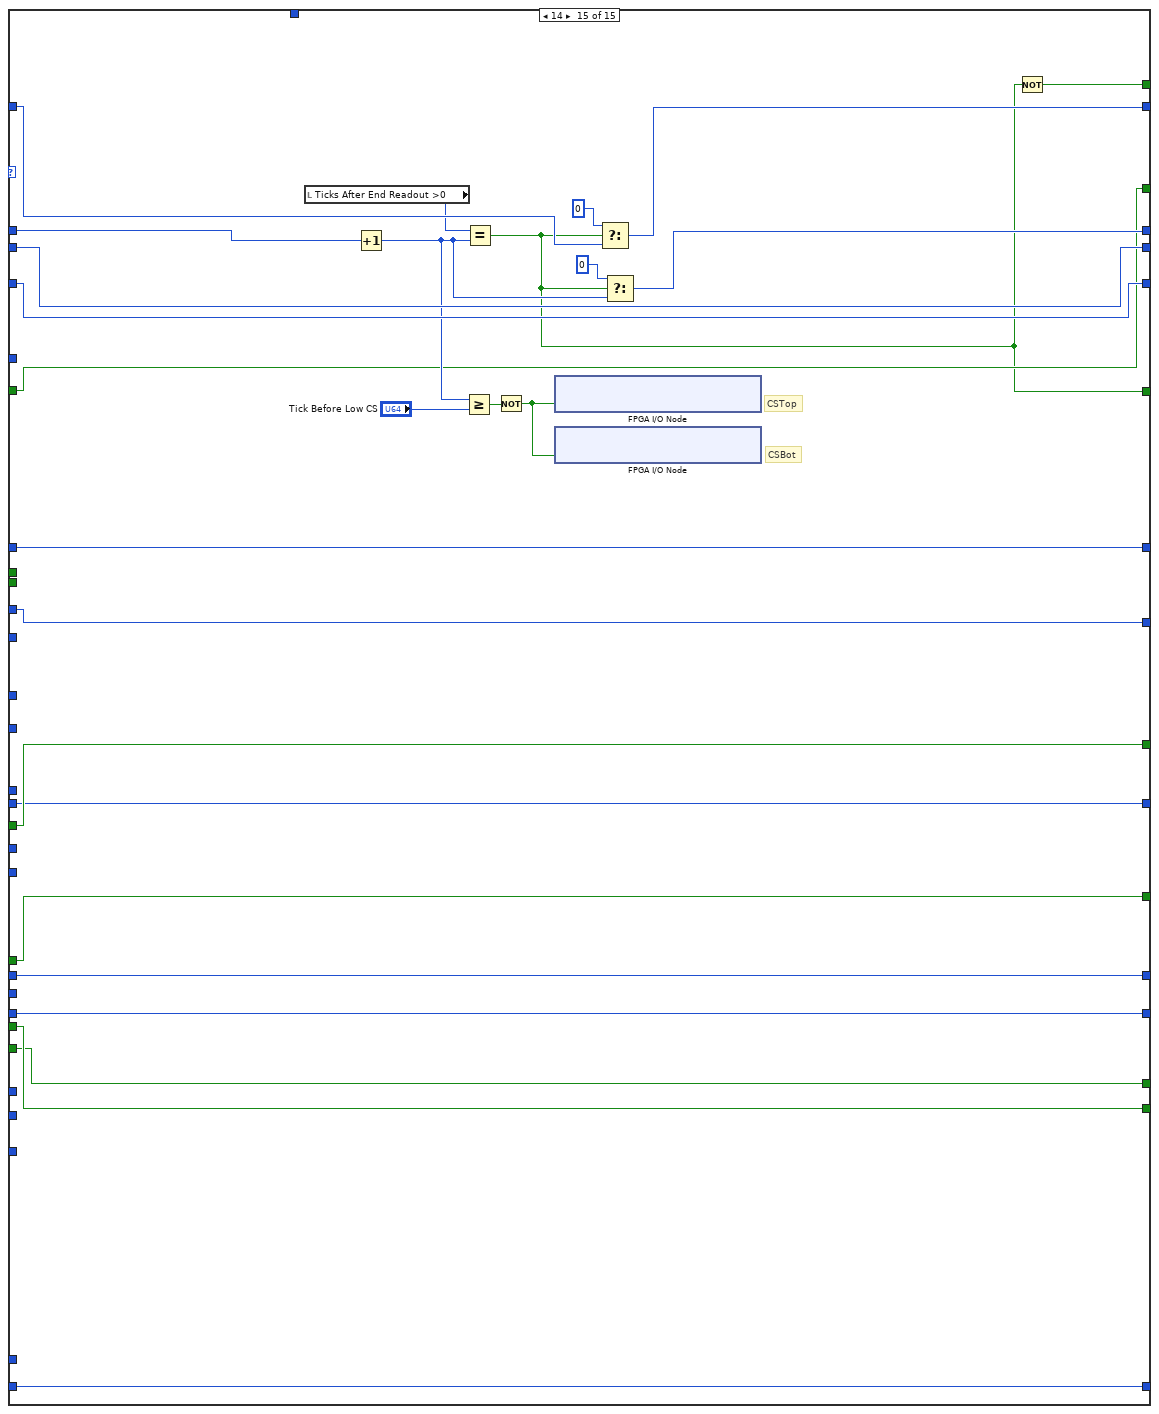
[diagram p20: hidden frame]
diagram:
  n1 = stacked-sequence {
    frame #0 {
      # "Логический уровень 3.3В"
      # "№\tDIO 16-23\tWE\n16\tP2.0\tCSTop\n17\tP2.1\tCmAD1\n18\tP2.2\tCmAD0\n19\tP2.3\tMCLK\n20\tP2.4\tCSBot\n21\tP2.5\tCmAD3\n22\tP2.6\tCmAD2\n23\tP2.7\tRS"
      # "№\tDIO 8-15\tWE\n8\tP1.0\tSLOAD\n9\tP1.1\tSCLK\n10\tP1.2\tCDSCLK2\n11\tP1.3\tCDSCLK1\n12\tP1.4\tADCCLK\n13\tP1.5\tIN1\n14\tP1.6\tIN2\n15\tP1.7-"
      # "PFI 1-3\tWE/RE\nPFI1\tSDATA\nPFI2\t-\nPFI3\t-"
      # "№\tDIO 0-7\tRE\n0\tP0.0\tD0\n1\tP0.1\tD1\n2\tP0.2\tD2\n3\tP0.3\tD3\n4\tP0.4\tD4\n5\tP0.5\tD5\n6\tP0.6\tD6\n7\tP0.7\tD7"
      # "Configure the power supply reference voltage"
      n2 = case shown="0, Default" "Supply Select" {
        frame 0, Default {
          w6 = u8 0 items=["3.3 Volts", "2.5 Volts", "1.8 Volts"] ("Internal Power Supply Voltage")
          n3 = xnode "FPGA I/O Node"("IO Module\\Local_Supply_Select"=w6) -> ()  [unwired: 1 in, 1 out]
        }
        frame 1 {
          n4 = xnode "FPGA I/O Node"("IO Module\\DDCA_Supply_Select"=TRUE ("IO Module\\DDCA_Supply_Select"), "IO Module\\DDCB_Supply_Select"=TRUE ("IO Module\\DDCB_Supply_Select")) -> ()  [unwired: 2 in, 2 out]
        }
      }
      n5 = xnode "FPGA I/O Node"("IO Module\\DDCA_DIO0-7_WE"=FALSE ("IO Module\\DDCA_DIO0-7_WE")) -> ()  [unwired: 1 in, 1 out]
      n6 = call "Wait"("Count(mSec)"=u8 10) -> ()  [unwired: 1 out]
      n7 = xnode "FPGA I/O Node"("IO Module\\DDCA_DIO8-15_WE"=TRUE ("IO Module\\DDCA_DIO8-15_WE")) -> ()  [unwired: 1 in, 1 out]
      n8 = xnode "FPGA I/O Node"("IO Module\\DDCA_DIO16-23_WE"=TRUE ("IO Module\\DDCA_DIO16-23_WE")) -> ()  [unwired: 1 in, 1 out]
    }
    frame #1 {
      w9 = FALSE
      n9 = node-c288() -> (w26:T2)  [unwired: 1 in]
      n10 = timed-loop {
        timing: w26 -> [_]
        timing-out: [_] -> w25
        shift-right: [w90] -> _
        shift-left: w9 -> [w70]
        shift-right: [w139] -> _
        shift-left: u8 0 -> [w141]
        shift-right: [w138] -> _
        shift-left: w9 -> [w135]
        shift-right: [w108] -> _
        shift-left: w9 -> [w107]
        shift-right: [w137] -> _
        shift-left: w9 -> [w91]
        shift-right: [w129] -> _
        shift-left: u8 0 -> [w122]
        shift-right: [w130] -> _
        shift-left: u8 0 -> [w123]
        shift-right: [w114] -> _
        shift-left: w9 -> [_]
        shift-right: [w113] -> _
        shift-left: u8 0 -> [w101]
        shift-right: [w95] -> _
        shift-left: u64 0 -> [w100]
        shift-right: [w96] -> _
        shift-left: u8 1 -> [w50]
        shift-right: [w93] -> _
        shift-left: u16 0 ("t") -> [w92]
        shift-right: [w86] -> _
        shift-left: u16 0 ("t") -> [w85]
        shift-right: [w83] -> _
        shift-left: w9 -> [w84]
        shift-right: [w78] -> _
        shift-left: u16 0 -> [w82]
        shift-right: [w79] -> _
        shift-left: u16 0 -> [w80]
        shift-right: [w71] -> _
        shift-left: w9 -> [w77]
        shift-right: [w74] -> _
        shift-left: w9 -> [w76]
        shift-right: [w72] -> _
        shift-left: u16 0 -> [w73]
        shift-right: [w63] -> _
        shift-left: u8 0 ("t") -> [w65]
        shift-right: [w60] -> _
        shift-left: w9 -> [w61]
        stop <- "Stop_FPGA" stop-if-true
        w49 = u8 4 ("x")
        w128 = u8 0 ("f")
        # "RS"
        # "Цикл: Спад - Фронт - Спад - Фронт"
        # "Конец передачи пары Command и Data, переход к следующей паре"
        # "Запуск по спаду (default) MCLK"
        # "Считать D7...D0 во время..."
        # "По спаду или фронту MCLK"
        # "Заземлен для  режима  1-Channel SHA Mode Timing"
        # "CDSCLK1"
        # "R 0 1 1 2\nF 1 1 2 2"
        # "Счетчик спадов CLK"
        # "Счетчик фронтов CLK"
        # "После 2-го фронта MCLK начало выдачи пикселей с линейки"
        # "На 3й фронт CDSCLK начало выдачи пикселей с АЦП"
        # "Отправить команду при количестве фронтов и спадов CLK"
        # "CLK (48 MHz)"
        # "1032 - количество пикселей Top и Bot с dummy\nGreen - Top, Blue - Bot\nИтого 4 адреса по 2 младших и страших 8 бит на 2 пикселя, 4128 адресов.\nОднако, в связи с ограничением принятия пикселей по частоте АЦП, можно принимать за раз либо Top, либо Bot. Итого 2064 адресов памяти\n\nNumberOfAdd = 2064"
        # "MCLK"
        n11 = Increment(x=w123) -> (x+1=w132:u8)
        n12 = Increment(x=w122) -> (x+1=w131:u8)
        n13 = Not(x=w107) -> (.not. x?=w133:bool)
        n14 = Select(t=w132, s=w107, f=w123) -> (s? t:f=w68:u8)
        n15 = Select(t=w131, s=w133, f=w122) -> (s? t:f=w69:u8)
        n16 = Not(x=w107) -> (.not. x?=w108:bool)
        n17 = xnode "FPGA I/O Node"("IO Module\\DDCA_DIO11_Write"=FALSE ("IO Module\\DDCA_DIO11_Write")) -> ()  [unwired: 1 in, 1 out]
        n18 = Equal?(x=w68, y="Rising CLK_1 = 0") -> (x = y?=w127:bool)
        n19 = Equal?(x=w69, y="Falling CLK_1 = 1") -> (x = y?=w124:bool)
        n20 = Not(x=w70) -> (.not. x?=w104:bool)
        n21 = And(x=w127, y=w124) -> (x .and. y?=w121:bool)
        n22 = Select(t=w104, s=w121, f=w70) -> (s? t:f=w136:bool)
        n23 = Add(x=w49, y=w50) -> (x+y=w56:u8)
        n24 = And(x="Автомат", y=w136) -> (x .and. y?=w90:bool)
        n25 = Less?(x=w50, y=w49) -> (x < y?=w52:bool)
        n26 = Equal?(x=w90, y="F(F)/R(T)_CmAD") -> (x = y?=w115:bool)
        n27 = Equal?(x=w68, y="Rising CLK_2 = 1") -> (x = y?=w117:bool)
        n28 = Equal?(x=w69, y="Falling CLK_2 = 2") -> (x = y?=w116:bool)
        n29 = xnode "FPGA I/O Node"("IO Module\\DDCA_DIO19_Write"=w90) -> ()  [unwired: 1 in, 1 out]
        n30 = And(x="GetCapture", y=w52) -> (x .and. y?=w51:bool)
        n31 = Compound Arithmetic op=OR("SetPreCapture", "SetFull", "GetCapture") -> (w57:bool)
        n32 = Compound Arithmetic op=AND(w117, w116, w115) -> (w102:bool)
        n33 = Select(t=w56, s=w51, f=w50) -> (s? t:f=w55:u8)
        n34 = Select(t=w135, s=w135, f=w102) -> (s? t:f=w103:bool)
        n35 = Not(x=w91) -> (.not. x?=w134:bool)
        n36 = Compound Arithmetic op=AND(w103, w134, w57) -> (w99:bool)
        n37 = Select(t=w55, s=w99, f=u8 0) -> (s? t:f=w97:u8)
        n38 = case shown="11" w97 {
          tunnel: w141 -> [w159 w202 w236 w288 w322 w371 w403 w452 w484 w533 w565 w627 w703 w752 w790]
          tunnel: [w159 w201 w236 w287 w322 w370 w403 w451 w484 w532 w565 w627 w703 w751 w790] -> w139
          tunnel: [w157 TRUE TRUE TRUE TRUE TRUE TRUE TRUE TRUE TRUE TRUE TRUE TRUE TRUE w772] -> w138
          tunnel: [w160 FALSE ("t") FALSE ("t") w247 FALSE ("t") FALSE ("t") FALSE ("t") FALSE ("t") FALSE ("t") FALSE ("t") FALSE ("t") FALSE ("t") FALSE ("t") FALSE ("t") w773] -> w137
          tunnel: w91 -> [w161 _ w227 _ w311 _ w391 _ w472 _ w553 w600 w700 _ w783]
          tunnel: [w157 w191 w227 w277 w311 w360 w391 w441 w472 w522 w553 w600 w700 w741 w783] -> w114
          tunnel: w101 -> [w158 w192 w237 w278 w323 w361 w404 w442 w485 w523 w566 w628 w704 w742 w791]
          tunnel: [w158 w195 w237 w281 w323 w364 w404 w445 w485 w526 w566 w628 w704 w745 w791] -> w113
          tunnel: "Counter R&F CLK_1 = 7" -> [_ w196 _ w282 _ w365 _ w446 _ w527 _ _ _ w746 _]
          tunnel: "Counter R&F CLK_2 = 4" -> [_ w193 _ w279 _ w362 _ w443 _ w524 _ _ _ w743 _]
          tunnel: w100 -> [_ w177 w234 w265 w320 w346 w401 w427 w482 w499 w563 w626 w701 w724 w789]
          tunnel: w55 -> [_ w185 w244 w271 w330 w354 w411 w435 w492 w516 w573 w606 w711 w735 w796]
          tunnel: [u8 1 w181 w243 w250 w329 w350 w410 w431 w491 w512 w572 w607 w710 w731 w795] -> w96
          tunnel: [u64 0 ("t") w177 w238 w265 w324 w346 w405 w427 w486 w499 w567 w626 w705 w724 w792] -> w95
          tunnel: "R MCLK = 2" -> [_ _ _ _ _ _ _ _ _ _ _ w643 _ _ _]
          tunnel: [u16 0 ("t") w175 w225 w263 w318 w344 w399 w425 w480 w508 w561 w605 w692 w727 w774] -> w93
          tunnel: w92 -> [_ w175 w225 w263 w318 w344 w399 w425 w480 w508 w561 w642 w692 w727 w774]
          tunnel: w90 -> [_ _ _ _ _ _ _ _ _ _ _ w625 _ _ _]
          tunnel: w70 -> [_ _ _ _ _ _ _ _ _ _ _ w641 _ _ _]
          tunnel: "1032 pixels" -> [_ _ _ _ _ _ _ _ _ _ _ w588 _ _ _]
          tunnel: "True ADCCLK Start = 1" -> [_ _ _ _ _ _ _ _ _ _ _ w640 _ _ _]
          tunnel: "True ADCCLK Stop = 4" -> [_ _ _ _ _ _ _ _ _ _ _ w639 _ _ _]
          tunnel: [u16 0 ("t") w174 w224 w260 w317 w343 w397 w418 w478 w503 w560 w604 w693 w722 w780] -> w86
          tunnel: w85 -> [_ w174 w224 w260 w317 w343 w397 w418 w478 w503 w560 w638 w693 w722 w780]
          tunnel: w84 -> [_ w173 w229 w262 w316 w342 w398 w424 w479 w504 w559 w637 w694 w721 w782]
          tunnel: [FALSE w173 w229 w262 w316 w342 w398 w424 w479 w504 w559 w636 w694 w721 w782] -> w83
          tunnel: w82 -> [_ w171 w230 w257 w314 w340 w394 w421 w475 w507 w557 w635 w696 w726 w779]
          tunnel: "Pixel (n-3) = 3" -> [_ _ _ _ _ _ _ _ _ _ _ w634 _ _ _]
          tunnel: w80 -> [_ w170 w231 w258 w313 w339 w393 w420 w474 w506 w556 w587 w697 w725 w778]
          tunnel: [u16 0 ("t") w170 w231 w258 w313 w339 w393 w420 w474 w506 w556 w602 w697 w725 w778] -> w79
          tunnel: [u16 0 ("t") w171 w230 w257 w314 w340 w394 w421 w475 w507 w557 w603 w696 w726 w779] -> w78
          tunnel: w77 -> [_ w172 w228 w261 w315 w341 w396 w423 w477 w502 w558 w633 w695 w720 w781]
          tunnel: w76 -> [_ w169 w232 w259 w310 w338 w395 w422 w476 w501 w555 w632 w698 w719 w777]
          tunnel: "Output Data _ADCCLK(T) = 3" -> [_ _ _ _ _ _ _ _ _ _ _ w631 _ _ _]
          tunnel: [FALSE w169 w232 w259 w310 w338 w395 w422 w476 w501 w555 w630 w698 w719 w777] -> w74
          tunnel: w73 -> [_ w168 w233 w256 w312 w337 w392 w419 w473 w500 w554 w629 w699 w718 w776]
          tunnel: [u16 0 ("t") w168 w233 w256 w312 w337 w392 w419 w473 w500 w554 w601 w699 w718 w776] -> w72
          tunnel: [FALSE w172 w228 w261 w315 w341 w396 w423 w477 w502 w558 w584 w695 w720 w781] -> w71
          tunnel: w65 -> [_ w176 w226 w264 w319 w345 w400 w426 w481 w505 w562 w578 w691 w723 w775]
          tunnel: "True CDSCLK2 Start = 4" -> [_ _ _ _ _ _ _ _ _ _ _ w623 _ _ _]
          tunnel: "True CDSCLK2 Stop = 5" -> [_ _ _ _ _ _ _ _ _ _ _ w620 _ _ _]
          tunnel: [u8 0 ("f") w176 w226 w264 w319 w345 w400 w426 w481 w505 w562 w612 w691 w723 w775] -> w63
          tunnel: "Output Data _ADCCLK(F) = 7" -> [_ _ _ _ _ _ _ _ _ _ _ w615 _ _ _]
          tunnel: w61 -> [_ w164 w223 w253 w309 w333 w390 w414 w471 w495 w552 w580 _ w714 w771]
          tunnel: [FALSE w164 w223 w253 w309 w333 w390 w414 w471 w495 w552 w583 FALSE w714 w771] -> w60
          tunnel: "FIFO Enable = 0" -> [_ _ _ _ _ _ _ _ _ _ _ w577 _ _ _]
          tunnel: "NumberOfAddFIFO" -> [_ _ _ _ _ _ _ _ _ _ _ w576 _ _ _]
          frame 0, Default {
            (unwired) FALSE ("f")
            w156 = FALSE ("t")
            w157 = FALSE
            # "CSTop"
            # "CSBot"
            # "CmAD3"
            # "CmAD2"
            # "CmAD1"
            # "CmAD0"
            n39 = xnode "FPGA I/O Node"("IO Module\\DDCA_DIO16_Write"=FALSE ("IO Module\\DDCA_DIO16_Write")) -> ()  [unwired: 1 in, 1 out]
            n40 = xnode "FPGA I/O Node"("IO Module\\DDCA_DIO18_Write"=w156) -> ()  [unwired: 1 in, 1 out]
            n41 = xnode "FPGA I/O Node"("IO Module\\DDCA_DIO17_Write"=w156) -> ()  [unwired: 1 in, 1 out]
            n42 = xnode "FPGA I/O Node"("IO Module\\DDCA_DIO22_Write"=w156) -> ()  [unwired: 1 in, 1 out]
            n43 = xnode "FPGA I/O Node"("IO Module\\DDCA_DIO21_Write"=w156) -> ()  [unwired: 1 in, 1 out]
            n44 = xnode "FPGA I/O Node"("IO Module\\DDCA_DIO20_Write"=FALSE ("IO Module\\DDCA_DIO20_Write")) -> ()  [unwired: 1 in, 1 out]
            n45 = Select(t=FALSE, s="ResetFrame", f=w161) -> (s? t:f=w160:bool)
          }
          frame 1 {
            # "CSTop"
            # "CSBot"
            # "Момент смены\nCommand на Data"
            # "Иммитация спада для повторного запуска кейса"
            # "Счетчик номера элемента массива"
            # "CmAD3"
            # "CmAD2"
            # "CmAD1"
            # "CmAD0"
            n46 = local read "Data CSTop"() -> (w190:u8[])
            n47 = local read "Command CS"() -> (w187:u8[])
            n48 = Greater Or Equal?(x=w192, y=w193) -> (x >= y?=w191:bool)
            n49 = Array Size(array=w187) -> (size(s)=w178:i32)
            n50 = Select(t=w190, s=w191, f=w187) -> (s? t:f=w218:u8[])
            n51 = To Long Integer(number=w202) -> (32bit integer=w217:i32)
            n52 = Increment(x=w202) -> (x+1=w220:u8)
            n53 = Index Array(array=w218, index=w217) -> (element=w219:u8)
            n54 = Less Or Equal?(x=w196, y=w192) -> (x <= y?=w198:bool)
            n55 = xnode "FPGA I/O Node"("IO Module\\DDCA_DIO16_Write"=TRUE ("IO Module\\DDCA_DIO16_Write")) -> ()  [unwired: 1 in, 1 out]
            n56 = To Long Integer(number=u8 0 ("CmAD0_bit_0")) -> (32bit integer=w207:i32)
            n57 = To Long Integer(number=u8 1 ("CmAD1_bit_1")) -> (32bit integer=w206:i32)
            n58 = To Long Integer(number=u8 2 ("CmAD2_bit_2")) -> (32bit integer=w205:i32)
            n59 = To Long Integer(number=u8 3 ("CmAD3_bit_3")) -> (32bit integer=w203:i32)
            n60 = Number To Boolean Array(number=w219) -> (Boolean array=w215:bool[])
            n61 = Select(t=w220, s=w198, f=w202) -> (s? t:f=w200:u8)
            n62 = Increment(x=w192) -> (x+1=w194:u8)
            n63 = Index Array(array=w215, index=w207) -> (element=w216:bool)
            n64 = Index Array(array=w215, index=w206) -> (element=w212:bool)
            n65 = Index Array(array=w215, index=w205) -> (element=w214:bool)
            n66 = Index Array(array=w215, index=w203) -> (element=w213:bool)
            n67 = Select(t=u8 0, s=w198, f=w194) -> (s? t:f=w195:u8)
            n68 = xnode "FPGA I/O Node"("IO Module\\DDCA_DIO18_Write"=w216) -> ()  [unwired: 1 in, 1 out]
            n69 = xnode "FPGA I/O Node"("IO Module\\DDCA_DIO17_Write"=w212) -> ()  [unwired: 1 in, 1 out]
            n70 = xnode "FPGA I/O Node"("IO Module\\DDCA_DIO22_Write"=w214) -> ()  [unwired: 1 in, 1 out]
            n71 = xnode "FPGA I/O Node"("IO Module\\DDCA_DIO21_Write"=w213) -> ()  [unwired: 1 in, 1 out]
            n72 = xnode "FPGA I/O Node"("IO Module\\DDCA_DIO20_Write"=FALSE ("IO Module\\DDCA_DIO20_Write")) -> ()  [unwired: 1 in, 1 out]
            n73 = To Unsigned Byte Integer(number=w178) -> (unsigned 8bit integer=w179:u8)
            n74 = Equal?(x=w200, y=w179) -> (x = y?=w165:bool)
            n75 = Select(t=u8 0, s=w165, f=w200) -> (s? t:f=w201:u8)
            n76 = Increment(x=w185) -> (x+1=w186:u8)
            n77 = Select(t=w186, s=w165, f=w185) -> (s? t:f=w183:u8)
            n78 = Equal To 0?(x="Ticks After Top >0") -> (x = 0?=w166:bool)
            n79 = Increment(x=w183) -> (x+1=w184:u8)
            n80 = And(x=w166, y=w165) -> (x .and. y?=w167:bool)
            n81 = Select(t=w184, s=w167, f=w183) -> (s? t:f=w181:u8)
          }
          frame 2 {
            # "CSTop"
            # "CSBot"
            n82 = xnode "FPGA I/O Node"("IO Module\\DDCA_DIO16_Write"=FALSE ("IO Module\\DDCA_DIO16_Write")) -> ()  [unwired: 1 in, 1 out]
            n83 = local read "Ticks After Top >0"() -> (w241:u64)
            n84 = Increment(x=w234) -> (x+1=w235:u64)
            n85 = Equal?(x=w241, y=w235) -> (x = y?=w239:bool)
            n86 = Increment(x=w244) -> (x+1=w245:u8)
            n87 = Select(t=w245, s=w239, f=w244) -> (s? t:f=w243:u8)
            n88 = xnode "FPGA I/O Node"("IO Module\\DDCA_DIO20_Write"=FALSE ("IO Module\\DDCA_DIO20_Write")) -> ()  [unwired: 1 in, 1 out]
            n89 = Select(t=u64 0, s=w239, f=w235) -> (s? t:f=w238:u64)
          }
          frame 3 {
            # "CSTop"
            # "CSBot"
            # "Момент смены\nCommand на Data"
            # "Иммитация спада для повторного запуска кейса"
            # "Счетчик номера элемента массива"
            # "CmAD3"
            # "CmAD2"
            # "CmAD1"
            # "CmAD0"
            n90 = local read "Data CSBot"() -> (w276:u8[])
            n91 = local read "Command CS"() -> (w273:u8[])
            n92 = Greater Or Equal?(x=w278, y=w279) -> (x >= y?=w277:bool)
            n93 = Array Size(array=w273) -> (size(s)=w266:i32)
            n94 = Select(t=w276, s=w277, f=w273) -> (s? t:f=w304:u8[])
            n95 = To Long Integer(number=w288) -> (32bit integer=w303:i32)
            n96 = Increment(x=w288) -> (x+1=w306:u8)
            n97 = Index Array(array=w304, index=w303) -> (element=w305:u8)
            n98 = Less Or Equal?(x=w282, y=w278) -> (x <= y?=w284:bool)
            n99 = xnode "FPGA I/O Node"("IO Module\\DDCA_DIO16_Write"=FALSE ("IO Module\\DDCA_DIO16_Write")) -> ()  [unwired: 1 in, 1 out]
            n100 = To Long Integer(number=u8 0 ("CmAD0_bit_0")) -> (32bit integer=w293:i32)
            n101 = To Long Integer(number=u8 1 ("CmAD1_bit_1")) -> (32bit integer=w292:i32)
            n102 = To Long Integer(number=u8 2 ("CmAD2_bit_2")) -> (32bit integer=w291:i32)
            n103 = To Long Integer(number=u8 3 ("CmAD3_bit_3")) -> (32bit integer=w289:i32)
            n104 = Number To Boolean Array(number=w305) -> (Boolean array=w301:bool[])
            n105 = Select(t=w306, s=w284, f=w288) -> (s? t:f=w286:u8)
            n106 = Increment(x=w278) -> (x+1=w280:u8)
            n107 = Index Array(array=w301, index=w293) -> (element=w302:bool)
            n108 = Index Array(array=w301, index=w292) -> (element=w298:bool)
            n109 = Index Array(array=w301, index=w291) -> (element=w300:bool)
            n110 = Index Array(array=w301, index=w289) -> (element=w299:bool)
            n111 = Select(t=u8 0, s=w284, f=w280) -> (s? t:f=w281:u8)
            n112 = xnode "FPGA I/O Node"("IO Module\\DDCA_DIO18_Write"=w302) -> ()  [unwired: 1 in, 1 out]
            n113 = xnode "FPGA I/O Node"("IO Module\\DDCA_DIO17_Write"=w298) -> ()  [unwired: 1 in, 1 out]
            n114 = xnode "FPGA I/O Node"("IO Module\\DDCA_DIO22_Write"=w300) -> ()  [unwired: 1 in, 1 out]
            n115 = xnode "FPGA I/O Node"("IO Module\\DDCA_DIO21_Write"=w299) -> ()  [unwired: 1 in, 1 out]
            n116 = xnode "FPGA I/O Node"("IO Module\\DDCA_DIO20_Write"=TRUE ("IO Module\\DDCA_DIO20_Write")) -> ()  [unwired: 1 in, 1 out]
            n117 = To Unsigned Byte Integer(number=w266) -> (unsigned 8bit integer=w267:u8)
            n118 = Equal?(x=w286, y=w267) -> (x = y?=w248:bool)
            n119 = Select(t=u8 0, s=w248, f=w286) -> (s? t:f=w287:u8)
            n120 = Increment(x=w271) -> (x+1=w272:u8)
            n121 = Select(t=w272, s=w248, f=w271) -> (s? t:f=w269:u8)
            n122 = local read "SetPreCapture"() -> (w249:bool)
            n123 = Equal To 0?(x="Ticks After Bot >0") -> (x = 0?=w254:bool)
            n124 = Increment(x=w269) -> (x+1=w270:u8)
            n125 = And(x=w254, y=w248) -> (x .and. y?=w255:bool)
            n126 = And(x=w249, y=w248) -> (x .and. y?=w247:bool)
            n127 = Select(t=w270, s=w255, f=w269) -> (s? t:f=w251:u8)
            n128 = Select(t=u8 0, s=w247, f=w251) -> (s? t:f=w250:u8)
          }
          frame 4 {
            # "CSTop"
            # "CSBot"
            n129 = local read "Ticks After Bot >0"() -> (w327:u64)
            n130 = xnode "FPGA I/O Node"("IO Module\\DDCA_DIO16_Write"=FALSE ("IO Module\\DDCA_DIO16_Write")) -> ()  [unwired: 1 in, 1 out]
            n131 = Increment(x=w320) -> (x+1=w321:u64)
            n132 = Equal?(x=w327, y=w321) -> (x = y?=w325:bool)
            n133 = Increment(x=w330) -> (x+1=w331:u8)
            n134 = Select(t=w331, s=w325, f=w330) -> (s? t:f=w329:u8)
            n135 = Select(t=u64 0, s=w325, f=w321) -> (s? t:f=w324:u64)
            n136 = xnode "FPGA I/O Node"("IO Module\\DDCA_DIO20_Write"=FALSE ("IO Module\\DDCA_DIO20_Write")) -> ()  [unwired: 1 in, 1 out]
          }
          frame 5 {
            # "CSTop"
            # "CSBot"
            # "Момент смены\nCommand на Data"
            # "Иммитация спада для повторного запуска кейса"
            # "Счетчик номера элемента массива"
            # "CmAD3"
            # "CmAD2"
            # "CmAD1"
            # "CmAD0"
            n137 = local read "Data Reset"() -> (w359:u8[])
            n138 = local read "Command Reset"() -> (w356:u8[])
            n139 = Greater Or Equal?(x=w361, y=w362) -> (x >= y?=w360:bool)
            n140 = Array Size(array=w356) -> (size(s)=w347:i32)
            n141 = Select(t=w359, s=w360, f=w356) -> (s? t:f=w387:u8[])
            n142 = To Long Integer(number=w371) -> (32bit integer=w386:i32)
            n143 = Increment(x=w371) -> (x+1=w389:u8)
            n144 = Index Array(array=w387, index=w386) -> (element=w388:u8)
            n145 = Less Or Equal?(x=w365, y=w361) -> (x <= y?=w367:bool)
            n146 = xnode "FPGA I/O Node"("IO Module\\DDCA_DIO16_Write"=TRUE ("IO Module\\DDCA_DIO16_Write")) -> ()  [unwired: 1 in, 1 out]
            n147 = To Long Integer(number=u8 0 ("CmAD0_bit_0")) -> (32bit integer=w376:i32)
            n148 = To Long Integer(number=u8 1 ("CmAD1_bit_1")) -> (32bit integer=w375:i32)
            n149 = To Long Integer(number=u8 2 ("CmAD2_bit_2")) -> (32bit integer=w374:i32)
            n150 = To Long Integer(number=u8 3 ("CmAD3_bit_3")) -> (32bit integer=w372:i32)
            n151 = Number To Boolean Array(number=w388) -> (Boolean array=w384:bool[])
            n152 = Select(t=w389, s=w367, f=w371) -> (s? t:f=w369:u8)
            n153 = Increment(x=w361) -> (x+1=w363:u8)
            n154 = Index Array(array=w384, index=w376) -> (element=w385:bool)
            n155 = Index Array(array=w384, index=w375) -> (element=w381:bool)
            n156 = Index Array(array=w384, index=w374) -> (element=w383:bool)
            n157 = Index Array(array=w384, index=w372) -> (element=w382:bool)
            n158 = Select(t=u8 0, s=w367, f=w363) -> (s? t:f=w364:u8)
            n159 = xnode "FPGA I/O Node"("IO Module\\DDCA_DIO18_Write"=w385) -> ()  [unwired: 1 in, 1 out]
            n160 = xnode "FPGA I/O Node"("IO Module\\DDCA_DIO17_Write"=w381) -> ()  [unwired: 1 in, 1 out]
            n161 = xnode "FPGA I/O Node"("IO Module\\DDCA_DIO22_Write"=w383) -> ()  [unwired: 1 in, 1 out]
            n162 = xnode "FPGA I/O Node"("IO Module\\DDCA_DIO21_Write"=w382) -> ()  [unwired: 1 in, 1 out]
            n163 = xnode "FPGA I/O Node"("IO Module\\DDCA_DIO20_Write"=TRUE ("IO Module\\DDCA_DIO20_Write")) -> ()  [unwired: 1 in, 1 out]
            n164 = To Unsigned Byte Integer(number=w347) -> (unsigned 8bit integer=w348:u8)
            n165 = Equal?(x=w369, y=w348) -> (x = y?=w334:bool)
            n166 = Select(t=u8 0, s=w334, f=w369) -> (s? t:f=w370:u8)
            n167 = Increment(x=w354) -> (x+1=w355:u8)
            n168 = Select(t=w355, s=w334, f=w354) -> (s? t:f=w352:u8)
            n169 = Equal To 0?(x="Ticks After Reset") -> (x = 0?=w335:bool)
            n170 = Increment(x=w352) -> (x+1=w353:u8)
            n171 = And(x=w335, y=w334) -> (x .and. y?=w336:bool)
            n172 = Select(t=w353, s=w336, f=w352) -> (s? t:f=w350:u8)
          }
          frame 6 {
            n173 = local read "Ticks After Reset"() -> (w408:u64)
            n174 = Increment(x=w401) -> (x+1=w402:u64)
            n175 = Equal?(x=w408, y=w402) -> (x = y?=w406:bool)
            n176 = Increment(x=w411) -> (x+1=w412:u8)
            n177 = Select(t=w412, s=w406, f=w411) -> (s? t:f=w410:u8)
            n178 = Select(t=u64 0, s=w406, f=w402) -> (s? t:f=w405:u64)
          }
          frame 7 {
            # "CSTop"
            # "CSBot"
            # "Момент смены\nCommand на Data"
            # "Иммитация спада для повторного запуска кейса"
            # "Счетчик номера элемента массива"
            # "CmAD3"
            # "CmAD2"
            # "CmAD1"
            # "CmAD0"
            n179 = local read "Data Start Integration"() -> (w440:u8[])
            n180 = local read "Command Start Integration"() -> (w437:u8[])
            n181 = Greater Or Equal?(x=w442, y=w443) -> (x >= y?=w441:bool)
            n182 = Array Size(array=w437) -> (size(s)=w428:i32)
            n183 = Select(t=w440, s=w441, f=w437) -> (s? t:f=w468:u8[])
            n184 = To Long Integer(number=w452) -> (32bit integer=w467:i32)
            n185 = Increment(x=w452) -> (x+1=w470:u8)
            n186 = Index Array(array=w468, index=w467) -> (element=w469:u8)
            n187 = Less Or Equal?(x=w446, y=w442) -> (x <= y?=w448:bool)
            n188 = xnode "FPGA I/O Node"("IO Module\\DDCA_DIO16_Write"=TRUE ("IO Module\\DDCA_DIO16_Write")) -> ()  [unwired: 1 in, 1 out]
            n189 = To Long Integer(number=u8 0 ("CmAD0_bit_0")) -> (32bit integer=w457:i32)
            n190 = To Long Integer(number=u8 1 ("CmAD1_bit_1")) -> (32bit integer=w456:i32)
            n191 = To Long Integer(number=u8 2 ("CmAD2_bit_2")) -> (32bit integer=w455:i32)
            n192 = To Long Integer(number=u8 3 ("CmAD3_bit_3")) -> (32bit integer=w453:i32)
            n193 = Number To Boolean Array(number=w469) -> (Boolean array=w465:bool[])
            n194 = Select(t=w470, s=w448, f=w452) -> (s? t:f=w450:u8)
            n195 = Increment(x=w442) -> (x+1=w444:u8)
            n196 = Index Array(array=w465, index=w457) -> (element=w466:bool)
            n197 = Index Array(array=w465, index=w456) -> (element=w462:bool)
            n198 = Index Array(array=w465, index=w455) -> (element=w464:bool)
            n199 = Index Array(array=w465, index=w453) -> (element=w463:bool)
            n200 = Select(t=u8 0, s=w448, f=w444) -> (s? t:f=w445:u8)
            n201 = xnode "FPGA I/O Node"("IO Module\\DDCA_DIO18_Write"=w466) -> ()  [unwired: 1 in, 1 out]
            n202 = xnode "FPGA I/O Node"("IO Module\\DDCA_DIO17_Write"=w462) -> ()  [unwired: 1 in, 1 out]
            n203 = xnode "FPGA I/O Node"("IO Module\\DDCA_DIO22_Write"=w464) -> ()  [unwired: 1 in, 1 out]
            n204 = xnode "FPGA I/O Node"("IO Module\\DDCA_DIO21_Write"=w463) -> ()  [unwired: 1 in, 1 out]
            n205 = xnode "FPGA I/O Node"("IO Module\\DDCA_DIO20_Write"=TRUE ("IO Module\\DDCA_DIO20_Write")) -> ()  [unwired: 1 in, 1 out]
            n206 = To Unsigned Byte Integer(number=w428) -> (unsigned 8bit integer=w429:u8)
            n207 = Equal?(x=w450, y=w429) -> (x = y?=w415:bool)
            n208 = Select(t=u8 0, s=w415, f=w450) -> (s? t:f=w451:u8)
            n209 = Increment(x=w435) -> (x+1=w436:u8)
            n210 = Select(t=w436, s=w415, f=w435) -> (s? t:f=w433:u8)
            n211 = Equal To 0?(x="Ticks After Start Integration") -> (x = 0?=w416:bool)
            n212 = Increment(x=w433) -> (x+1=w434:u8)
            n213 = And(x=w416, y=w415) -> (x .and. y?=w417:bool)
            n214 = Select(t=w434, s=w417, f=w433) -> (s? t:f=w431:u8)
          }
          frame 8 {
            n215 = local read "Ticks After Start Integration"() -> (w489:u64)
            n216 = Increment(x=w482) -> (x+1=w483:u64)
            n217 = Equal?(x=w489, y=w483) -> (x = y?=w487:bool)
            n218 = Increment(x=w492) -> (x+1=w493:u8)
            n219 = Select(t=w493, s=w487, f=w492) -> (s? t:f=w491:u8)
            n220 = Select(t=u64 0, s=w487, f=w483) -> (s? t:f=w486:u64)
          }
          frame 9 {
            # "CSTop"
            # "CSBot"
            # "Момент смены\nCommand на Data"
            # "Иммитация спада для повторного запуска кейса"
            # "Счетчик номера элемента массива"
            # "CmAD3"
            # "CmAD2"
            # "CmAD1"
            # "CmAD0"
            n221 = local read "Data Start Readout"() -> (w521:u8[])
            n222 = local read "Command Start Readout"() -> (w518:u8[])
            n223 = Greater Or Equal?(x=w523, y=w524) -> (x >= y?=w522:bool)
            n224 = Array Size(array=w518) -> (size(s)=w509:i32)
            n225 = Select(t=w521, s=w522, f=w518) -> (s? t:f=w549:u8[])
            n226 = To Long Integer(number=w533) -> (32bit integer=w548:i32)
            n227 = Increment(x=w533) -> (x+1=w551:u8)
            n228 = Index Array(array=w549, index=w548) -> (element=w550:u8)
            n229 = Less Or Equal?(x=w527, y=w523) -> (x <= y?=w529:bool)
            n230 = xnode "FPGA I/O Node"("IO Module\\DDCA_DIO16_Write"=TRUE ("IO Module\\DDCA_DIO16_Write")) -> ()  [unwired: 1 in, 1 out]
            n231 = To Long Integer(number=u8 0 ("CmAD0_bit_0")) -> (32bit integer=w538:i32)
            n232 = To Long Integer(number=u8 1 ("CmAD1_bit_1")) -> (32bit integer=w537:i32)
            n233 = To Long Integer(number=u8 2 ("CmAD2_bit_2")) -> (32bit integer=w536:i32)
            n234 = To Long Integer(number=u8 3 ("CmAD3_bit_3")) -> (32bit integer=w534:i32)
            n235 = Number To Boolean Array(number=w550) -> (Boolean array=w546:bool[])
            n236 = Select(t=w551, s=w529, f=w533) -> (s? t:f=w531:u8)
            n237 = Increment(x=w523) -> (x+1=w525:u8)
            n238 = Index Array(array=w546, index=w538) -> (element=w547:bool)
            n239 = Index Array(array=w546, index=w537) -> (element=w543:bool)
            n240 = Index Array(array=w546, index=w536) -> (element=w545:bool)
            n241 = Index Array(array=w546, index=w534) -> (element=w544:bool)
            n242 = Select(t=u8 0, s=w529, f=w525) -> (s? t:f=w526:u8)
            n243 = xnode "FPGA I/O Node"("IO Module\\DDCA_DIO18_Write"=w547) -> ()  [unwired: 1 in, 1 out]
            n244 = xnode "FPGA I/O Node"("IO Module\\DDCA_DIO17_Write"=w543) -> ()  [unwired: 1 in, 1 out]
            n245 = xnode "FPGA I/O Node"("IO Module\\DDCA_DIO22_Write"=w545) -> ()  [unwired: 1 in, 1 out]
            n246 = xnode "FPGA I/O Node"("IO Module\\DDCA_DIO21_Write"=w544) -> ()  [unwired: 1 in, 1 out]
            n247 = xnode "FPGA I/O Node"("IO Module\\DDCA_DIO20_Write"=TRUE ("IO Module\\DDCA_DIO20_Write")) -> ()  [unwired: 1 in, 1 out]
            n248 = To Unsigned Byte Integer(number=w509) -> (unsigned 8bit integer=w510:u8)
            n249 = Equal?(x=w531, y=w510) -> (x = y?=w496:bool)
            n250 = Select(t=u8 0, s=w496, f=w531) -> (s? t:f=w532:u8)
            n251 = Increment(x=w516) -> (x+1=w517:u8)
            n252 = Select(t=w517, s=w496, f=w516) -> (s? t:f=w514:u8)
            n253 = Equal To 0?(x="Ticks After Start Readout") -> (x = 0?=w497:bool)
            n254 = Increment(x=w514) -> (x+1=w515:u8)
            n255 = And(x=w497, y=w496) -> (x .and. y?=w498:bool)
            n256 = Select(t=w515, s=w498, f=w514) -> (s? t:f=w512:u8)
          }
          frame 10 {
            n257 = local read "Ticks After Start Readout"() -> (w570:u64)
            n258 = Increment(x=w563) -> (x+1=w564:u64)
            n259 = Equal?(x=w570, y=w564) -> (x = y?=w568:bool)
            n260 = Increment(x=w573) -> (x+1=w574:u8)
            n261 = Select(t=w574, s=w568, f=w573) -> (s? t:f=w572:u8)
            n262 = Select(t=u64 0, s=w568, f=w564) -> (s? t:f=w567:u64)
          }
          frame 11 {
            # "Счетчик тиков от начала работы кадра"
            # "Счетчик фронтов FIFO"
            # "ADCCLK"
            # "Счетчик спадов CDSCLK2"
            # "Счетчик фронтов ADCCLK"
            # "Счетчик фронтов MCLK"
            # "D7"
            # "D6"
            # "D5"
            # "D4"
            # "D3"
            # "D2"
            # "D1"
            # "D0"
            # "CDSCLK2"
            n263 = Less?(x=w578, y=w640) -> (x < y?=w617:bool)
            n264 = Greater?(x=w578, y=w639) -> (0:w616:bool)
            n265 = Less?(x=w578, y=w623) -> (x < y?=w622:bool)
            n266 = Greater?(x=w578, y=w620) -> (0:w621:bool)
            n267 = Equal?(x=w578, y=w631) -> (x = y?=w614:bool)
            n268 = Equal?(x=w578, y=w615) -> (x = y?=w613:bool)
            n269 = Greater?(x=w625, y=w641) -> (0:w657:bool)
            n270 = Increment(x=w642) -> (x+1=w654:u16)
            n271 = Less?(x=w638, y=w588) -> (x < y?=w660:bool)
            n272 = Not Or(1:w616, 2:w617) -> (0:w618:bool)
            n273 = Not Or(1:w621, 2:w622) -> (0:w624:bool)
            n274 = Select(t=w654, s=w657, f=w642) -> (s? t:f=w605:u16)
            n275 = xnode "FPGA I/O Node"() -> ("IO Module\\DDCA_DIO0_Read"=w652:bool, "IO Module\\DDCA_DIO1_Read"=w651:bool, "IO Module\\DDCA_DIO2_Read"=w650:bool, "IO Module\\DDCA_DIO3_Read"=w649:bool, "IO Module\\DDCA_DIO4_Read"=w648:bool, "IO Module\\DDCA_DIO5_Read"=w647:bool, "IO Module\\DDCA_DIO6_Read"=w646:bool, "IO Module\\DDCA_DIO7_Read"=w645:bool)  [unwired: 8 in, 8 out]
            n276 = Greater Or Equal?(x=w605, y=w643) -> (x >= y?=w664:bool)
            n277 = Less?(x=w587, y=w576) -> (x < y?=w661:bool)
            n278 = Compound Arithmetic op=AND(w664, w624, w660) -> (w636:bool)
            n279 = Increment(x=w638) -> (x+1=w656:u16)
            n280 = Compound Arithmetic op=AND(w618, w661) -> (w584:bool)
            n281 = Less?(x=w636, y=w637) -> (x < y?=w658:bool)
            n282 = Increment(x=w635) -> (x+1=w655:u16)
            n283 = Greater?(x=w584, y=w633) -> (0:w659:bool)
            n284 = Equal?(x="Ticks Reset = 7", y=w578) -> (x = y?=w619:bool)
            n285 = Increment(x=w578) -> (x+1=w593:u8)
            n286 = Or(x=w614, y=w613) -> (x .or. y?=w582:bool)
            n287 = Select(t=w656, s=w658, f=w638) -> (s? t:f=w604:u16)
            n288 = Select(t=w655, s=w659, f=w635) -> (s? t:f=w603:u16)
            n289 = case shown="False" "7..0(F)/0..7(T)" {
              tunnel: w652 -> [w674 w682]
              tunnel: w651 -> [w673 w681]
              tunnel: w650 -> [w672 w680]
              tunnel: w649 -> [w671 w679]
              tunnel: w648 -> [w670 w678]
              tunnel: w647 -> [w669 w677]
              tunnel: w646 -> [w668 w676]
              tunnel: w645 -> [w667 w675]
              tunnel: [w665 w683] -> w653
              frame False {
                n290 = Build Array(w674, w673, w672, w671, w670, w669, w668, w667) -> (w666:bool[])
                n291 = Boolean Array To Number(Boolean array=w666) -> (number=w665:u8)
              }
              frame True {
                n292 = Build Array(w675, w676, w677, w678, w679, w680, w681, w682) -> (w684:bool[])
                n293 = Boolean Array To Number(Boolean array=w684) -> (number=w683:u8)
              }
            }
            n294 = Select(t=u8 0 ("f"), s=w619, f=w593) -> (s? t:f=w612:u8)
            n295 = Equal?(x=w578, y=w577) -> (x = y?=w579:bool)
            n296 = Greater Or Equal?(x=w604, y=w634) -> (x >= y?=w585:bool)
            n297 = xnode "FPGA I/O Node"("IO Module\\DDCA_DIO10_Write"=w636) -> ()  [unwired: 1 in, 1 out]
            n298 = And(x=w585, y=w579) -> (x .and. y?=w581:bool)
            n299 = Select(t=w580, s=w580, f=w581) -> (s? t:f=w583:bool)
            n300 = xnode "FPGA I/O Node"("IO Module\\DDCA_DIO12_Write"=w584) -> ()  [unwired: 1 in, 1 out]
            n301 = Less?(x=w587, y=w576) -> (x < y?=w586:bool)
            n302 = Compound Arithmetic op=AND(w586, w583, w582) -> (w630:bool)
            n303 = case shown="True" w630 {
              tunnel: [w685 w689] -> w601
              tunnel: w629 -> [w685 w688]
              tunnel: w653 -> [_ w686]
              frame False {
              }
              frame True {
                n304 = Increment(x=w688) -> (x+1=w689:u16)
                n305 = xnode ("FIFO Method Node")("Element"=w686, "Timeout"=0) -> ()  [unwired: 1 in, 2 out]
              }
            }
            "FIFOCounter" <- w601
            n306 = Greater?(x=w632, y=w630) -> (0:w662:bool)
            n307 = Increment(x=w587) -> (x+1=w663:u16)
            n308 = Select(t=w663, s=w662, f=w587) -> (s? t:f=w602:u16)
            n309 = Equal?(x="Stop FIFO Frame", y=w578) -> (x = y?=w591:bool)
            n310 = Equal?(x=w576, y=w601) -> (x = y?=w590:bool)
            n311 = And(x=w591, y=w590) -> (x .and. y?=w589:bool)
            n312 = Increment(x=w606) -> (x+1=w611:u8)
            n313 = Select(t=w611, s=w589, f=w606) -> (s? t:f=w609:u8)
            n314 = Equal To 0?(x="Ticks After ADC") -> (x = 0?=w596:bool)
            n315 = Increment(x=w609) -> (x+1=w610:u8)
            n316 = And(x=w596, y=w589) -> (x .and. y?=w597:bool)
            n317 = Select(t=w610, s=w597, f=w609) -> (s? t:f=w607:u8)
          }
          frame 12 {
            n318 = local read "Ticks After ADC"() -> (w708:u64)
            n319 = Increment(x=w701) -> (x+1=w702:u64)
            n320 = Equal?(x=w708, y=w702) -> (x = y?=w706:bool)
            n321 = Increment(x=w711) -> (x+1=w712:u8)
            n322 = Select(t=w712, s=w706, f=w711) -> (s? t:f=w710:u8)
            n323 = Select(t=u64 0, s=w706, f=w702) -> (s? t:f=w705:u64)
          }
          frame 13 {
            # "CSTop"
            # "CSBot"
            # "Момент смены\nCommand на Data"
            # "Иммитация спада для повторного запуска кейса"
            # "Счетчик номера элемента массива"
            # "CmAD3"
            # "CmAD2"
            # "CmAD1"
            # "CmAD0"
            n324 = local read "Data End Readout"() -> (w740:u8[])
            n325 = local read "Command End Readout"() -> (w737:u8[])
            n326 = Greater Or Equal?(x=w742, y=w743) -> (x >= y?=w741:bool)
            n327 = Array Size(array=w737) -> (size(s)=w728:i32)
            n328 = Select(t=w740, s=w741, f=w737) -> (s? t:f=w768:u8[])
            n329 = To Long Integer(number=w752) -> (32bit integer=w767:i32)
            n330 = Increment(x=w752) -> (x+1=w770:u8)
            n331 = Index Array(array=w768, index=w767) -> (element=w769:u8)
            n332 = Less Or Equal?(x=w746, y=w742) -> (x <= y?=w748:bool)
            n333 = xnode "FPGA I/O Node"("IO Module\\DDCA_DIO16_Write"=TRUE ("IO Module\\DDCA_DIO16_Write")) -> ()  [unwired: 1 in, 1 out]
            n334 = To Long Integer(number=u8 0 ("CmAD0_bit_0")) -> (32bit integer=w757:i32)
            n335 = To Long Integer(number=u8 1 ("CmAD1_bit_1")) -> (32bit integer=w756:i32)
            n336 = To Long Integer(number=u8 2 ("CmAD2_bit_2")) -> (32bit integer=w755:i32)
            n337 = To Long Integer(number=u8 3 ("CmAD3_bit_3")) -> (32bit integer=w753:i32)
            n338 = Number To Boolean Array(number=w769) -> (Boolean array=w765:bool[])
            n339 = Select(t=w770, s=w748, f=w752) -> (s? t:f=w750:u8)
            n340 = Increment(x=w742) -> (x+1=w744:u8)
            n341 = Index Array(array=w765, index=w757) -> (element=w766:bool)
            n342 = Index Array(array=w765, index=w756) -> (element=w762:bool)
            n343 = Index Array(array=w765, index=w755) -> (element=w764:bool)
            n344 = Index Array(array=w765, index=w753) -> (element=w763:bool)
            n345 = Select(t=u8 0, s=w748, f=w744) -> (s? t:f=w745:u8)
            n346 = xnode "FPGA I/O Node"("IO Module\\DDCA_DIO18_Write"=w766) -> ()  [unwired: 1 in, 1 out]
            n347 = xnode "FPGA I/O Node"("IO Module\\DDCA_DIO17_Write"=w762) -> ()  [unwired: 1 in, 1 out]
            n348 = xnode "FPGA I/O Node"("IO Module\\DDCA_DIO22_Write"=w764) -> ()  [unwired: 1 in, 1 out]
            n349 = xnode "FPGA I/O Node"("IO Module\\DDCA_DIO21_Write"=w763) -> ()  [unwired: 1 in, 1 out]
            n350 = xnode "FPGA I/O Node"("IO Module\\DDCA_DIO20_Write"=TRUE ("IO Module\\DDCA_DIO20_Write")) -> ()  [unwired: 1 in, 1 out]
            n351 = To Unsigned Byte Integer(number=w728) -> (unsigned 8bit integer=w729:u8)
            n352 = Equal?(x=w750, y=w729) -> (x = y?=w715:bool)
            n353 = Select(t=u8 0, s=w715, f=w750) -> (s? t:f=w751:u8)
            n354 = Increment(x=w735) -> (x+1=w736:u8)
            n355 = Select(t=w736, s=w715, f=w735) -> (s? t:f=w733:u8)
            n356 = Equal To 0?(x="Ticks After End Readout >0") -> (x = 0?=w716:bool)
            n357 = Increment(x=w733) -> (x+1=w734:u8)
            n358 = And(x=w716, y=w715) -> (x .and. y?=w717:bool)
            n359 = Select(t=w734, s=w717, f=w733) -> (s? t:f=w731:u8)
          }
          frame 14 {
            # "CSBot"
            # "CSTop"
            n360 = local read "Ticks After End Readout >0"() -> (w794:u64)
            n361 = Increment(x=w789) -> (x+1=w787:u64)
            n362 = Greater Or Equal?(x=w787, y="Tick Before Low CS") -> (x >= y?=w785:bool)
            n363 = Equal?(x=w794, y=w787) -> (x = y?=w773:bool)
            n364 = Not(x=w785) -> (.not. x?=w784:bool)
            n365 = xnode "FPGA I/O Node"("IO Module\\DDCA_DIO16_Write"=w784) -> ()  [unwired: 1 in, 1 out]
            n366 = xnode "FPGA I/O Node"("IO Module\\DDCA_DIO20_Write"=w784) -> ()  [unwired: 1 in, 1 out]
            n367 = Select(t=u8 0, s=w773, f=w796) -> (s? t:f=w795:u8)
            n368 = Select(t=u64 0, s=w773, f=w787) -> (s? t:f=w792:u64)
            n369 = Not(x=w773) -> (.not. x?=w772:bool)
          }
        }
        "FrameIsDone" <- w137
        n370 = xnode "FPGA I/O Node"("IO Module\\DDCA_DIO23_Write"="RS") -> ()  [unwired: 1 in, 1 out]
        n371 = Equal?(x="Counter R CLK = 2", y=w68) -> (x = y?=w105:bool)
        n372 = Select(t=w128, s=w105, f=w68) -> (s? t:f=w130:u8)
        n373 = Select(t=w128, s=w105, f=w69) -> (s? t:f=w129:u8)
      }
      n374 = while {
        shift-right: ["Конфигурация"] -> _
        shift-left: FALSE ("Конфигурация") -> [w37]
        stop <- w34 stop-if-true
        n375 = Greater?(x="Конфигурация", y=w37) -> (0:w36:bool)
        n376 = case shown="True" w36 {
          frame False {
            n377 = call "Wait2"("Count(Ticks)"=u8 2) -> ()  [unwired: 1 out]
          }
          frame True {
            n378 = call "ADC_spb.vi"(1:"18_1"=i8 18 ("18_1"), 2:"18_1"=i8 18 ("18_1"), "8"=i8 8, "7"=i8 7, "Write Data"="Write Data", "Enum"="Enum", "Read(T)/Write(F)"="Read(T)/Write(F)", "Command array"="Command array") -> ("READ"=→"READ":bool[])
          }
        }
        n379 = local read "Stop_FPGA"() -> (w34:bool)
      }
      n380 = node-c288() -> (w20:T2)  [unwired: 1 in]
      n381 = timed-loop {
        timing: w20 -> [_]
        timing-out: [_] -> w19
        stop <- w27 stop-if-true
        # "IN1\tIN2\t\n\t0\t0\tOutTop_n\n\t0\t1\tOutTop_p\n\t1\t0\tOutBot_p\n\t1\t1\tOutBot_n"
        # "IN1"
        # "IN2"
        n382 = xnode "FPGA I/O Node"("IO Module\\DDCA_DIO13_Write"="IN1") -> ()  [unwired: 1 in, 1 out]
        n383 = xnode "FPGA I/O Node"("IO Module\\DDCA_DIO14_Write"="IN2") -> ()  [unwired: 1 in, 1 out]
        n384 = local read "Stop_FPGA"() -> (w27:bool)
      }
      n385 = node-c288(w19) -> ()
      n386 = node-c288(w25) -> ()
    }
  }
